vi "2D scan tiled.vi"(11 "Tiled scan inputs":T6={"HW Config"={"SEM X coil"="SEM-X", "SEM Y coil"="SEM-Y", "Detectors"="Detectors", "Det min (V)"=-10.0, "Det max (V)"=10.0, "Eanable COM"=TRUE, "COM port"="COM1", "Detector FIB-NI auto switch"="FIB/port0/line0", "Machine Type"=0, "Machine ID"="Feiss/Sigma-01-42"}, "Det Info"={"Brightness A"=40.0, "Contrast A"=26.0, "Detector B name"="ESB @ 1.0 kV", "Brightness B"=40.0, "Contrast B"=40.0, "Detector C name"="PMT @ 6.0", "Detector D name"="Detector D"}, "SEM Scan Parameters"={"X size (um)"=20.0, "Y size (um)"=20.0, "X center (um)"=0.0, "Y center (um)"=0.0, "X size (V)"=6.190428211586902, "X size auto"=TRUE, "X stig"=[[0.0]], "Y stig"=[[0.0]], "X aln"=[[0.0]], "Y aln"=[[0.0]], "Scan rate (Hz)"=10000000, "Oversampling"=5, "Oversampling auto"=TRUE, "Frame line rampdown ratio"=0.1, "Pixel size (nm)"=10.0, "WD (mm)"=[[3.0]], "X tiles"=1, "Y tiles"=1, "Overlap (um)"=1.0, "Interlaced"=TRUE, "dX (um)"=[0.0], "dY (um)"=[0.0], "Frames"=1}, "SEM Options"={"GetInfo"=TRUE, "Set Det A para"=TRUE, "Set WD"=FALSE, "Set Mag"=TRUE, "Set stig"=FALSE, "Set aln"=FALSE, "Display"=TRUE, "Save"=TRUE, "8-bit"=TRUE, "Detector A"=TRUE, "Detector B"=FALSE, "Detector C"=FALSE, "Detector D"=FALSE, "Inverse A"=FALSE, "Inverse B"=FALSE, "Inverse C"=FALSE, "Inverse D"=FALSE, "Inverse PNG"=TRUE, "Freeze"=TRUE, "PNG only"=FALSE, "Upload"=FALSE, "Delete after upload"=FALSE}, "Focus Index Options"={"Keep aspect ratio"=FALSE, "Show Focus Index"=TRUE, "Focus Index primary grid center"=TRUE, "X Grids"=[[0]], "Y Grids"=[[0]], "Primary X index"=[[0]], "Primary Y index"=[[0]]}, "File Information"={"File path"=path "E:/Images", "Notes"="", "Save recipe"=FALSE, "Load recipe"=FALSE, "Sample ID"=""}, "Milling para"={"X resolution"=4096, "Y resolution"=125001, "X offset (um)"=0.0, "Y offset (um)"=0.0, "X center (um)"=0.0, "Y center (um)"=0.0, "X size (um)"=250.0, "Y size (um)"=250.0, "UL-Ang"=90.0, "UR-Ang"=90.0, "Line milling time (s)"=5.0, "Z-step (nm)"=2.0, "Lines auto pause"=1, "Auto pause"=FALSE, "Mill from Bottom"=FALSE, "FIB FOV (um)"=500.0, "Auto Profile"=FALSE, "Mill start from Last"=FALSE, "FIB PID on"=FALSE, "FIB PID reset"=TRUE, "FIB PID measured"=0, "FIB PID target"=0.0, "FIB PID target slope"=0.0, "FIB PID P"=0.001, "FIB PID I"=0.01, "FIB PID D"=0.0, "Emission (uA)"=1.36, "Suppressor (V)"=50.0, "Auto reheat"=FALSE}} {"Milling para"."Suppressor (V)" step=0.1 format="%.1g"; "Milling para"."Emission (uA)" step=0.1 format="%.2g"; "Milling para"."FIB PID measured" items=["Spec.", "B.D. 1", "B.D. 2", "Mill", "Spec. +"]; "Milling para"."FIB PID target slope" min=-1 max=1 step=0.1; "Milling para"."UR-Ang" format="%.2f"; "Milling para"."UL-Ang" format="%.2f"; "Milling para"."Y offset (um)" step=0.02 format="%.3g"; "Milling para"."X offset (um)" step=1 format="%.3g"; "Milling para"."FIB FOV (um)" format="%.3g"; "Milling para"."Line milling time (s)" format="%.1f"; "Milling para"."Y center (um)" format="%#.3g"; "Milling para"."X center (um)" format="%#.3g"; "SEM Scan Parameters"."dY (um)" format="%.1f"; "SEM Scan Parameters"."dX (um)" format="%.1f"; "SEM Scan Parameters"."Frames" min=1 step=1; "SEM Scan Parameters"."WD (mm)" format="%.1f"; "SEM Scan Parameters"."Y aln" format="%.1f"; "SEM Scan Parameters"."X aln" format="%.1f"; "SEM Scan Parameters"."Y stig" format="%.1f"; "SEM Scan Parameters"."X stig" format="%.1f"; "SEM Scan Parameters"."Overlap (um)" min=0; "SEM Scan Parameters"."Y tiles" min=1; "SEM Scan Parameters"."X tiles" min=1; "SEM Scan Parameters"."X size (um)" format="%.2f"; "SEM Scan Parameters"."Y size (um)" format="%.2f"; "SEM Scan Parameters"."Frame line rampdown ratio" min=0 max=1 step=0.05 format="%.2g"; "SEM Scan Parameters"."X center (um)" step=1 format="%.2f"; "SEM Scan Parameters"."Y center (um)" step=1 format="%.2f"; "SEM Scan Parameters"."X size (V)" format="%_4g"; "SEM Scan Parameters"."Scan rate (Hz)" max=4000000 step=100000 format="%.2e"; "HW Config"."Machine Type" items=["Feiss", "NVision"]}) -> (0 "Image Focus Index Tiled":T3, 1 "Image Focus Index Array Tiled":T2, 2 "Low res scale Tiled (um/pix)":dbl[][](array[numeric]), 3 "Single scan outputs":T4={"SEM Status"={"AO SampClk.MaxRate"=100000000.0, "AI SampClk.MaxRate"=100000000.0, "AO rate"=10000000.0, "Scan speed"=1, "Detector #"=1, "X min (V)"=-3.095214105793451, "X max (V)"=3.095214105793451, "X min index"=0, "X max index"=1999, "AO multiline"=64, "Decimating factor"=3, "AvailSampPerChan"=832704, "AO scan line"=2000, "Total pixels recorded"=4096000, "Lines scanned"=2000, "Scan time (m)"=0.0, "Scan time (s)"=0.4416, "Remaining time (m)"=0, "Remaining time (s)"=0, "SEM Spec. I (nA)"=0.0, "Frame"=1, "X tile"=1, "Y tile"=1}, "SEM Parameters"={"Detector A"="InLens", "Detector B"="ESB @ 1.0 kV", "Brightness A"=40.0, "Contrast A"=26.0, "Brightness B"=40.0, "Contrast B"=40.0, "Magnification"=1769.4047, "Pixel size"=3.9210947, "Working distance"=2.91745, "EHT"=0.6, "Aperture"=1, "High current mode"=1, "Probe current"=613.0, "Scan rotation"=260.0, "Chamber vac"=1.43287e-06, "Gun vac"=3.9272e-10, "Beam shift X"=0.0, "Beam shift Y"=0.0, "Stig X"=-4.213583, "Stig Y"=-1.875912, "Alignment X"=1.861752, "Alignment Y"=-2.407838, "Stage X"=68.4182, "Stage Y"=64.91782, "Stage Z"=32.8349, "Stage T"=0.0, "Stage R"=153.14406, "Stage M"=0.0}, "Image Focus Index"={"A Img Focus Index"=0.014358657, "B Img Focus Index"=0.0, "C Img Focus Index"=0.0, "D Img Focus Index"=0.0}, "FIB parameters"={"FIB mode"=0, "FIB focus"=0.0, "FIB probe current"=0.0, "FIB emission current"=0.0, "FIB rotation"=0.0, "FIB aperture X"=0.0, "FIB aperture Y"=0.0, "FIB stig X"=0.0, "FIB stig Y"=0.0, "FIB beam shift X"=0.0, "FIB beam shift Y"=0.0}, "Image Focus Index Array"={"A Img Focus Index array"=[[0.014358657]], "B Img Focus Index array"=[], "C Img Focus Index array"=[], "D Img Focus Index array"=[]}} {"SEM Status"."Frame" min=1 step=1; "SEM Status"."Y tile" min=1; "SEM Status"."X tile" min=1; "SEM Status"."SEM Spec. I (nA)" format="%.2g"; "SEM Status"."AvailSampPerChan" scale=0.0..32000000.0; "SEM Status"."Scan time (s)" format="%.3f"; "SEM Status"."Total pixels recorded" scale=-1.0..37748736.0; "SEM Status"."Scan speed" scale=1.0..15.0; "SEM Status"."AO rate" format="%#_3e"}, 4 "SEM Spec. I Tiled (nA)":sgl[][](array[numeric]), 5 "8-bit over scale":bool[](array[boolean]))   [LabVIEW 2018]
uses:
  <vilib>/Analysis/baseanly.llb/Mean (DBL).vi
  <vilib>/Analysis/NI_AALBase.lvlib
panel:
  in  "Focus Index Options":T1={"Keep aspect ratio"=FALSE, "X Grids"=1, "Y Grids"=1, "Primary X index"=0, "Primary Y index"=0}
  in  "Api":refnum<k7>(container)
  out "Aln X Tiled":sgl[][](array[numeric])
  out "Aln Y Tiled":sgl[][](array[numeric])
  out "Stig Y Tiled":sgl[][](array[numeric])
  out "Stig X Tiled":sgl[][](array[numeric])
  out "WD Tiled":sgl[][](array[numeric])
  out "Det B Img Tiled":i16[][](graph)
  out "Det A Img Tiled":i16[][](graph)
  out "Tiled image Y index":u16[][](array[numeric])
  out "Tiled image X index":u16[][](array[numeric])
  out "Tiled image scale (um/pix)":sgl
  out "X size (V)":dbl[][](array[numeric])=[[2000.0]]
  out "Y center (um)":sgl[][](array[numeric])
  out "X center (um)":sgl[][](array[numeric])
  out "Y resolution":u32[][](array[numeric])=[[2000]]
  out "X resolution":u32[][](array[numeric])=[[2000]]
  in  "SEM Scan Parameters":T5={"X resolution"=6144, "Y resolution"=6144, "X center (um)"=0.0, "Y center (um)"=0.0, "X size (V)"=6.190428211586902, "X size auto"=TRUE, "X stig"=0.0, "Y stig"=0.0, "X aln"=0.0, "Y aln"=0.0, "Scan rate (Hz)"=10000000, "Oversampling"=5, "Oversampling auto"=TRUE, "Frame line rampdown ratio"=0.1, "Pixel size (nm)"=10.0, "WD (mm)"=0.0} {"Y aln" step=0.2 format="%.1g"; "X aln" step=0.2 format="%.1g"; "Y stig" step=0.2 format="%.1g"; "X stig" step=0.2 format="%.1g"; "WD (mm)" step=0.001 format="%.6g"; "Frame line rampdown ratio" min=0 max=1 step=0.05 format="%.2g"; "X center (um)" step=1.0 format="%.2f"; "Y center (um)" step=1.0 format="%.2f"; "X size (V)" format="%_4g"; "Scan rate (Hz)" max=4000000 step=100000 format="%.2e"}
  # "Hz"
  # "Scanning time"
  # "m"
  # "s"
  # "Remaining time"
  # "m"
  # "s"
  # "Direction"
  # "Start\nfrom"
  # "<"
  # "Grids"
  # "Primary"
  # "Recipe"
  # "Det"
  # "after"
  # "Detector A"
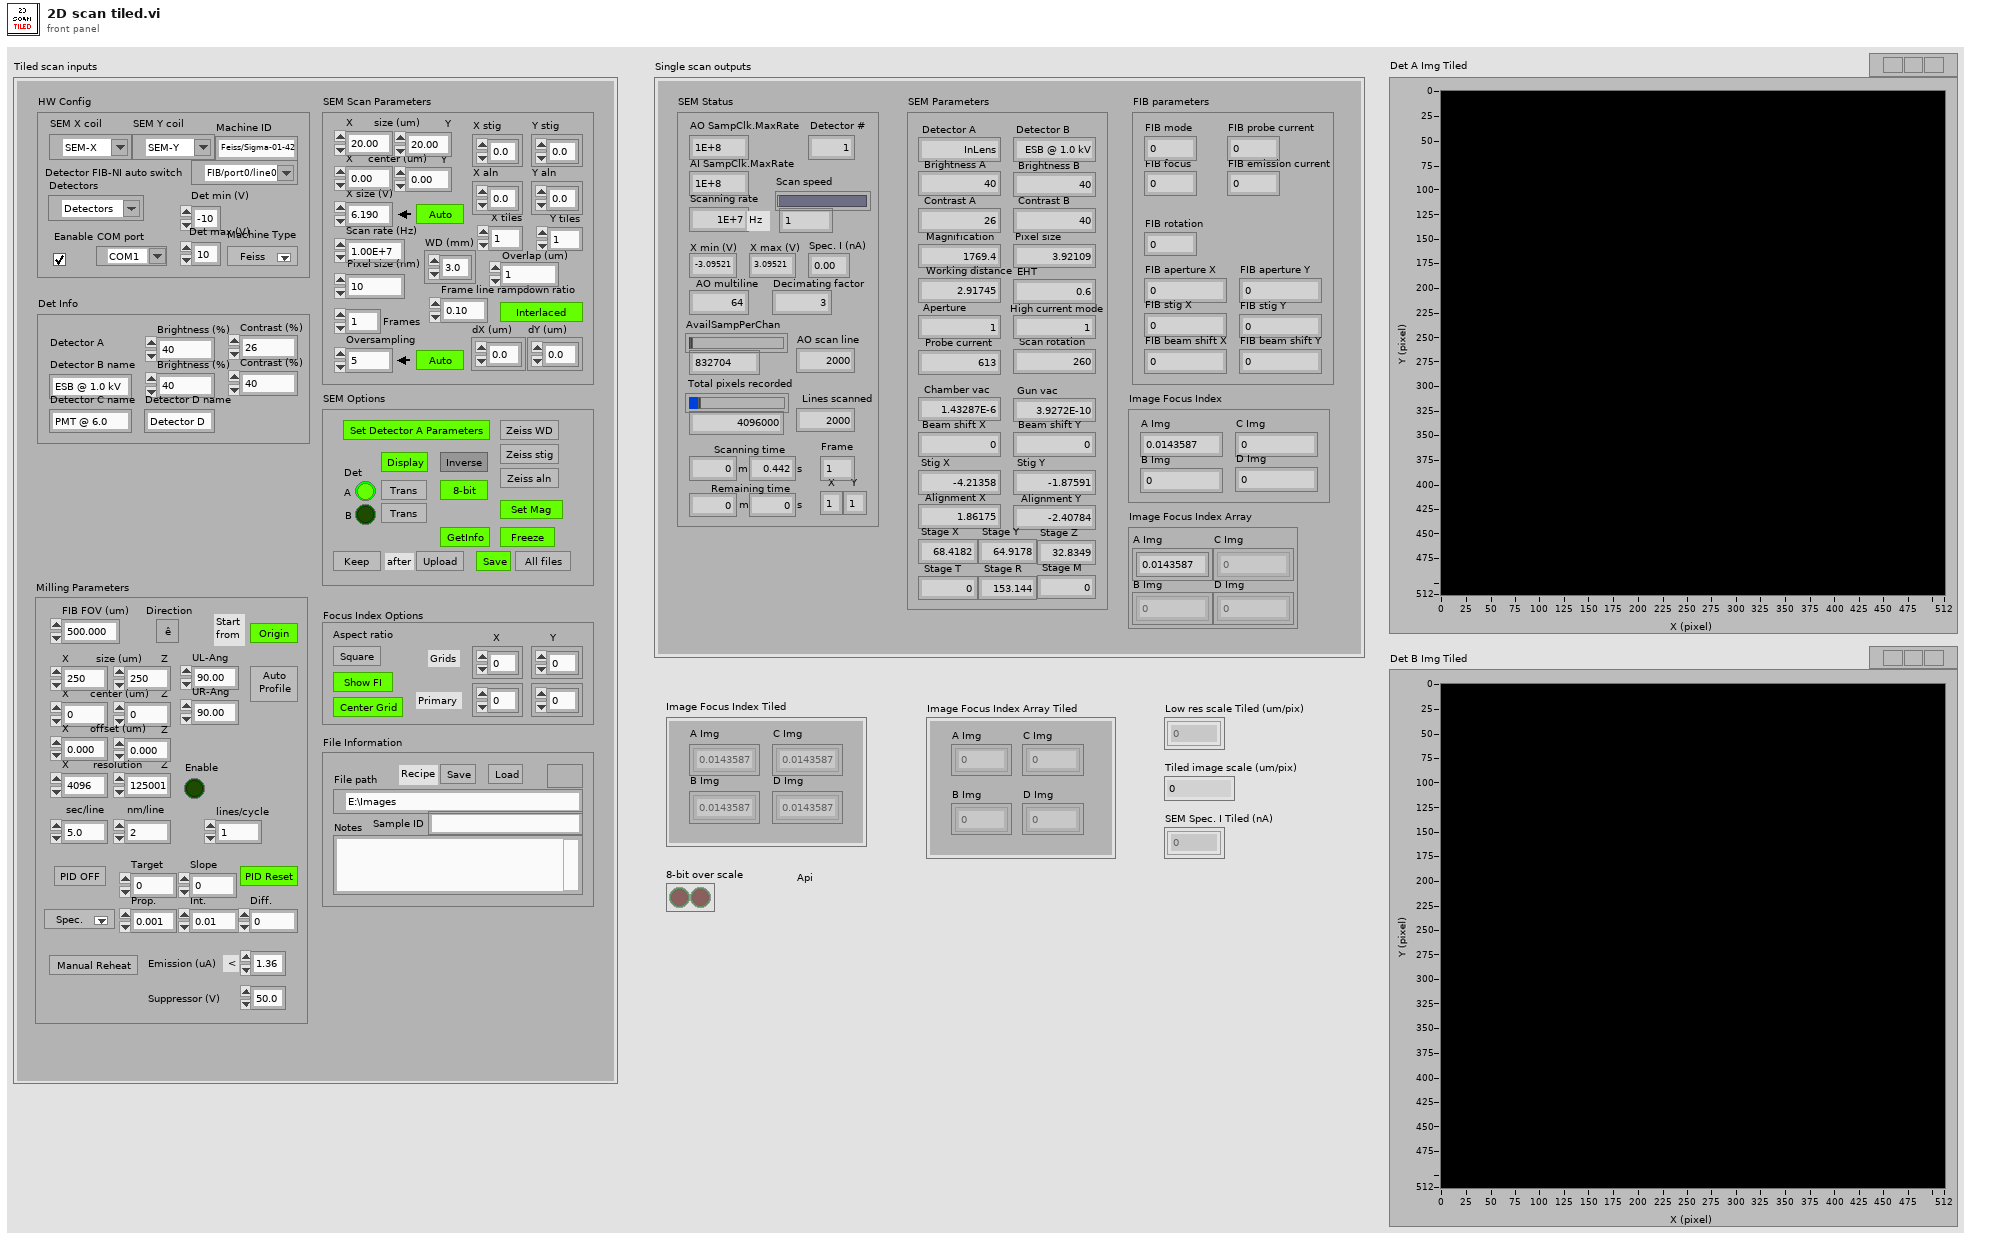
[diagram p1: front panel]
types:
  T1 = cluster{"Keep aspect ratio":bool, "X Grids":u8, "Y Grids":u8, "Primary X index":u8, "Primary Y index":u8}
  T2 = cluster{"A Img Focus Index array":sgl[][][][], "B Img Focus Index array":sgl[][][][], "C Img Focus Index array":sgl[][][][], "D Img Focus Index array":sgl[][][][]}
  T3 = cluster{"A Img Focus Index":sgl[][], "B Img Focus Index":sgl[][], "C Img Focus Index":sgl[][], "D Img Focus Index":sgl[][]}
  T4 = cluster{"SEM Status":cluster{"AO SampClk.MaxRate":dbl, "AI SampClk.MaxRate":dbl, "AO rate":dbl, "Scan speed":u8, "Detector #":u8, "X min (V)":dbl, "X max (V)":dbl, "X min index":i32, "X max index":i32, "AO multiline":u32, "Decimating factor":u16, "AvailSampPerChan":u32, "AO scan line":u32, "Total pixels recorded":i32, "Lines scanned":i32, "Scan time (m)":dbl, "Scan time (s)":dbl, "Remaining time (m)":u16, "Remaining time (s)":u8, "SEM Spec. I (nA)":sgl, "Frame":u8, "X tile":u8, "Y tile":u8}, "SEM Parameters":cluster{"Detector A":string, "Detector B":string, "Brightness A":sgl, "Contrast A":sgl, "Brightness B":sgl, "Contrast B":sgl, "Magnification":sgl, "Pixel size":sgl, "Working distance":sgl, "EHT":sgl, "Aperture":u8, "High current mode":u8, "Probe current":sgl, "Scan rotation":sgl, "Chamber vac":sgl, "Gun vac":sgl, "Beam shift X":sgl, "Beam shift Y":sgl, "Stig X":sgl, "Stig Y":sgl, "Alignment X":sgl, "Alignment Y":sgl, "Stage X":sgl, "Stage Y":sgl, "Stage Z":sgl, "Stage T":sgl, "Stage R":sgl, "Stage M":sgl}, "Image Focus Index":cluster{"A Img Focus Index":sgl, "B Img Focus Index":sgl, "C Img Focus Index":sgl, "D Img Focus Index":sgl}, "FIB parameters":cluster{"FIB mode":u8, "FIB focus":sgl, "FIB probe current":sgl, "FIB emission current":sgl, "FIB rotation":sgl, "FIB aperture X":sgl, "FIB aperture Y":sgl, "FIB stig X":sgl, "FIB stig Y":sgl, "FIB beam shift X":sgl, "FIB beam shift Y":sgl}, "Image Focus Index Array":cluster{"A Img Focus Index array":sgl[][], "B Img Focus Index array":sgl[][], "C Img Focus Index array":sgl[][], "D Img Focus Index array":sgl[][]}}
  T5 = cluster{"X resolution":u32, "Y resolution":u32, "X center (um)":dbl, "Y center (um)":dbl, "X size (V)":dbl, "X size auto":bool, "X stig":sgl, "Y stig":sgl, "X aln":sgl, "Y aln":sgl, "Scan rate (Hz)":u32, "Oversampling":u32, "Oversampling auto":bool, "Frame line rampdown ratio":sgl, "Pixel size (nm)":sgl, "WD (mm)":sgl}
  T6 = cluster{"HW Config":cluster{"SEM X coil":refnum<k15>, "SEM Y coil":refnum<k15>, "Detectors":refnum<k15>, "Det min (V)":dbl, "Det max (V)":dbl, "Eanable COM":bool, "COM port":refnum<visa-resource-name>, "Detector FIB-NI auto switch":tag, "Machine Type":u8, "Machine ID":string}, "Det Info":cluster{"Brightness A":dbl, "Contrast A":dbl, "Detector B name":string, "Brightness B":dbl, "Contrast B":dbl, "Detector C name":string, "Detector D name":string}, "SEM Scan Parameters":cluster{"X size (um)":sgl, "Y size (um)":sgl, "X center (um)":sgl, "Y center (um)":sgl, "X size (V)":dbl, "X size auto":bool, "X stig":sgl[][], "Y stig":sgl[][], "X aln":sgl[][], "Y aln":sgl[][], "Scan rate (Hz)":u32, "Oversampling":u32, "Oversampling auto":bool, "Frame line rampdown ratio":sgl, "Pixel size (nm)":sgl, "WD (mm)":sgl[][], "X tiles":u8, "Y tiles":u8, "Overlap (um)":sgl, "Interlaced":bool, "dX (um)":sgl[], "dY (um)":sgl[], "Frames":u8}, "SEM Options":cluster{"GetInfo":bool, "Set Det A para":bool, "Set WD":bool, "Set Mag":bool, "Set stig":bool, "Set aln":bool, "Display":bool, "Save":bool, "8-bit":bool, "Detector A":bool, "Detector B":bool, "Detector C":bool, "Detector D":bool, "Inverse A":bool, "Inverse B":bool, "Inverse C":bool, "Inverse D":bool, "Inverse PNG":bool, "Freeze":bool, "PNG only":bool, "Upload":bool, "Delete after upload":bool}, "Focus Index Options":cluster{"Keep aspect ratio":bool, "Show Focus Index":bool, "Focus Index primary grid center":bool, "X Grids":u8[][], "Y Grids":u8[][], "Primary X index":u8[][], "Primary Y index":u8[][]}, "File Information":cluster{"File path":path, "Notes":string, "Save recipe":bool, "Load recipe":bool, "Sample ID":string}, "Milling para":cluster{"X resolution":u32, "Y resolution":u32, "X offset (um)":sgl, "Y offset (um)":sgl, "X center (um)":sgl, "Y center (um)":sgl, "X size (um)":sgl, "Y size (um)":sgl, "UL-Ang":sgl, "UR-Ang":sgl, "Line milling time (s)":sgl, "Z-step (nm)":dbl, "Lines auto pause":u16, "Auto pause":bool, "Mill from Bottom":bool, "FIB FOV (um)":sgl, "Auto Profile":bool, "Mill start from Last":bool, "FIB PID on":bool, "FIB PID reset":bool, "FIB PID measured":u8, "FIB PID target":sgl, "FIB PID target slope":sgl, "FIB PID P":sgl, "FIB PID I":sgl, "FIB PID D":sgl, "Emission (uA)":dbl, "Suppressor (V)":sgl, "Auto reheat":bool}}
  T7 = cluster{"GetInfo":bool, "Set Det A para":bool, "Set WD":bool, "Set Mag":bool, "Set stig":bool, "Set aln":bool, "Display":bool, "Save":bool, "8-bit":bool, "Detector A":bool, "Detector B":bool, "Detector C":bool, "Detector D":bool, "Inverse A":bool, "Inverse B":bool, "Inverse C":bool, "Inverse D":bool, "Inverse PNG":bool, "Freeze":bool, "PNG only":bool, "Upload":bool, "Delete after upload":bool}
  T8 = cluster{"SEM X coil":refnum<k15>, "SEM Y coil":refnum<k15>, "Detectors":refnum<k15>, "Det min (V)":dbl, "Det max (V)":dbl, "Eanable COM":bool, "COM port":refnum<visa-resource-name>, "Detector FIB-NI auto switch":tag, "Machine Type":u8, "Machine ID":string}
  T9 = cluster{"Brightness A":dbl, "Contrast A":dbl, "Detector B name":string, "Brightness B":dbl, "Contrast B":dbl, "Detector C name":string, "Detector D name":string}
  T10 = cluster{"X size (um)":sgl, "Y size (um)":sgl, "X center (um)":sgl, "Y center (um)":sgl, "X size (V)":dbl, "X size auto":bool, "X stig":sgl[][], "Y stig":sgl[][], "X aln":sgl[][], "Y aln":sgl[][], "Scan rate (Hz)":u32, "Oversampling":u32, "Oversampling auto":bool, "Frame line rampdown ratio":sgl, "Pixel size (nm)":sgl, "WD (mm)":sgl[][], "X tiles":u8, "Y tiles":u8, "Overlap (um)":sgl, "Interlaced":bool, "dX (um)":sgl[], "dY (um)":sgl[], "Frames":u8}
  T11 = cluster{"Keep aspect ratio":bool, "Show Focus Index":bool, "Focus Index primary grid center":bool, "X Grids":u8[][], "Y Grids":u8[][], "Primary X index":u8[][], "Primary Y index":u8[][]}
  T12 = cluster{"File path":path, "Notes":string, "Save recipe":bool, "Load recipe":bool, "Sample ID":string}
  T13 = cluster{"X resolution":u32, "Y resolution":u32, "X offset (um)":sgl, "Y offset (um)":sgl, "X center (um)":sgl, "Y center (um)":sgl, "X size (um)":sgl, "Y size (um)":sgl, "UL-Ang":sgl, "UR-Ang":sgl, "Line milling time (s)":sgl, "Z-step (nm)":dbl, "Lines auto pause":u16, "Auto pause":bool, "Mill from Bottom":bool, "FIB FOV (um)":sgl, "Auto Profile":bool, "Mill start from Last":bool, "FIB PID on":bool, "FIB PID reset":bool, "FIB PID measured":u8, "FIB PID target":sgl, "FIB PID target slope":sgl, "FIB PID P":sgl, "FIB PID I":sgl, "FIB PID D":sgl, "Emission (uA)":dbl, "Suppressor (V)":sgl, "Auto reheat":bool}
  T14 = cluster{"A Img Focus Index array":sgl[][], "B Img Focus Index array":sgl[][], "C Img Focus Index array":sgl[][], "D Img Focus Index array":sgl[][]}
  T15 = cluster{"AO SampClk.MaxRate":dbl, "AI SampClk.MaxRate":dbl, "AO rate":dbl, "Scan speed":u8, "Detector number":u8, "X min (V)":dbl, "X max (V)":dbl, "X min index":i32, "X max index":i32, "AO multiline":u32, "Decimating factor":u16, "AvailSampPerChan":u32, "AO scan line":u32, "Total pixels recorded":i32, "Total lines scanned":i32, "Scan time (m)":dbl, "Scan time (s)":dbl, "Remaining time (m)":u16, "Remaining time (s)":u8, "Specimen I (nA)":sgl, "Frame":u8, "X tile":u8, "Y tile":u8}
  T16 = cluster{"Detector A":string, "Detector B":string, "Brightness A":sgl, "Contrast A":sgl, "Brightness B":sgl, "Contrast B":sgl, "Magnification":sgl, "Pixel size":sgl, "Working distance":sgl, "EHT":sgl, "Aperture":u8, "High current mode":u8, "Probe current":sgl, "Scan rotation":sgl, "Chamber vac":sgl, "Gun vac":sgl, "Beam shift X":sgl, "Beam shift Y":sgl, "Stig X":sgl, "Stig Y":sgl, "Alignment X":sgl, "Alignment Y":sgl, "Stage X":sgl, "Stage Y":sgl, "Stage Z":sgl, "Stage T":sgl, "Stage R":sgl, "Stage M":sgl}
  T17 = cluster{"FIB mode":u8, "FIB focus":sgl, "FIB probe current":sgl, "FIB emission current":sgl, "FIB rotation":sgl, "FIB aperture X":sgl, "FIB aperture Y":sgl, "FIB stig X":sgl, "FIB stig Y":sgl, "FIB beam shift X":sgl, "FIB beam shift Y":sgl}
  T18 = cluster{"A Img Focus Index":sgl, "B Img Focus Index":sgl, "C Img Focus Index":sgl, "D Img Focus Index":sgl}
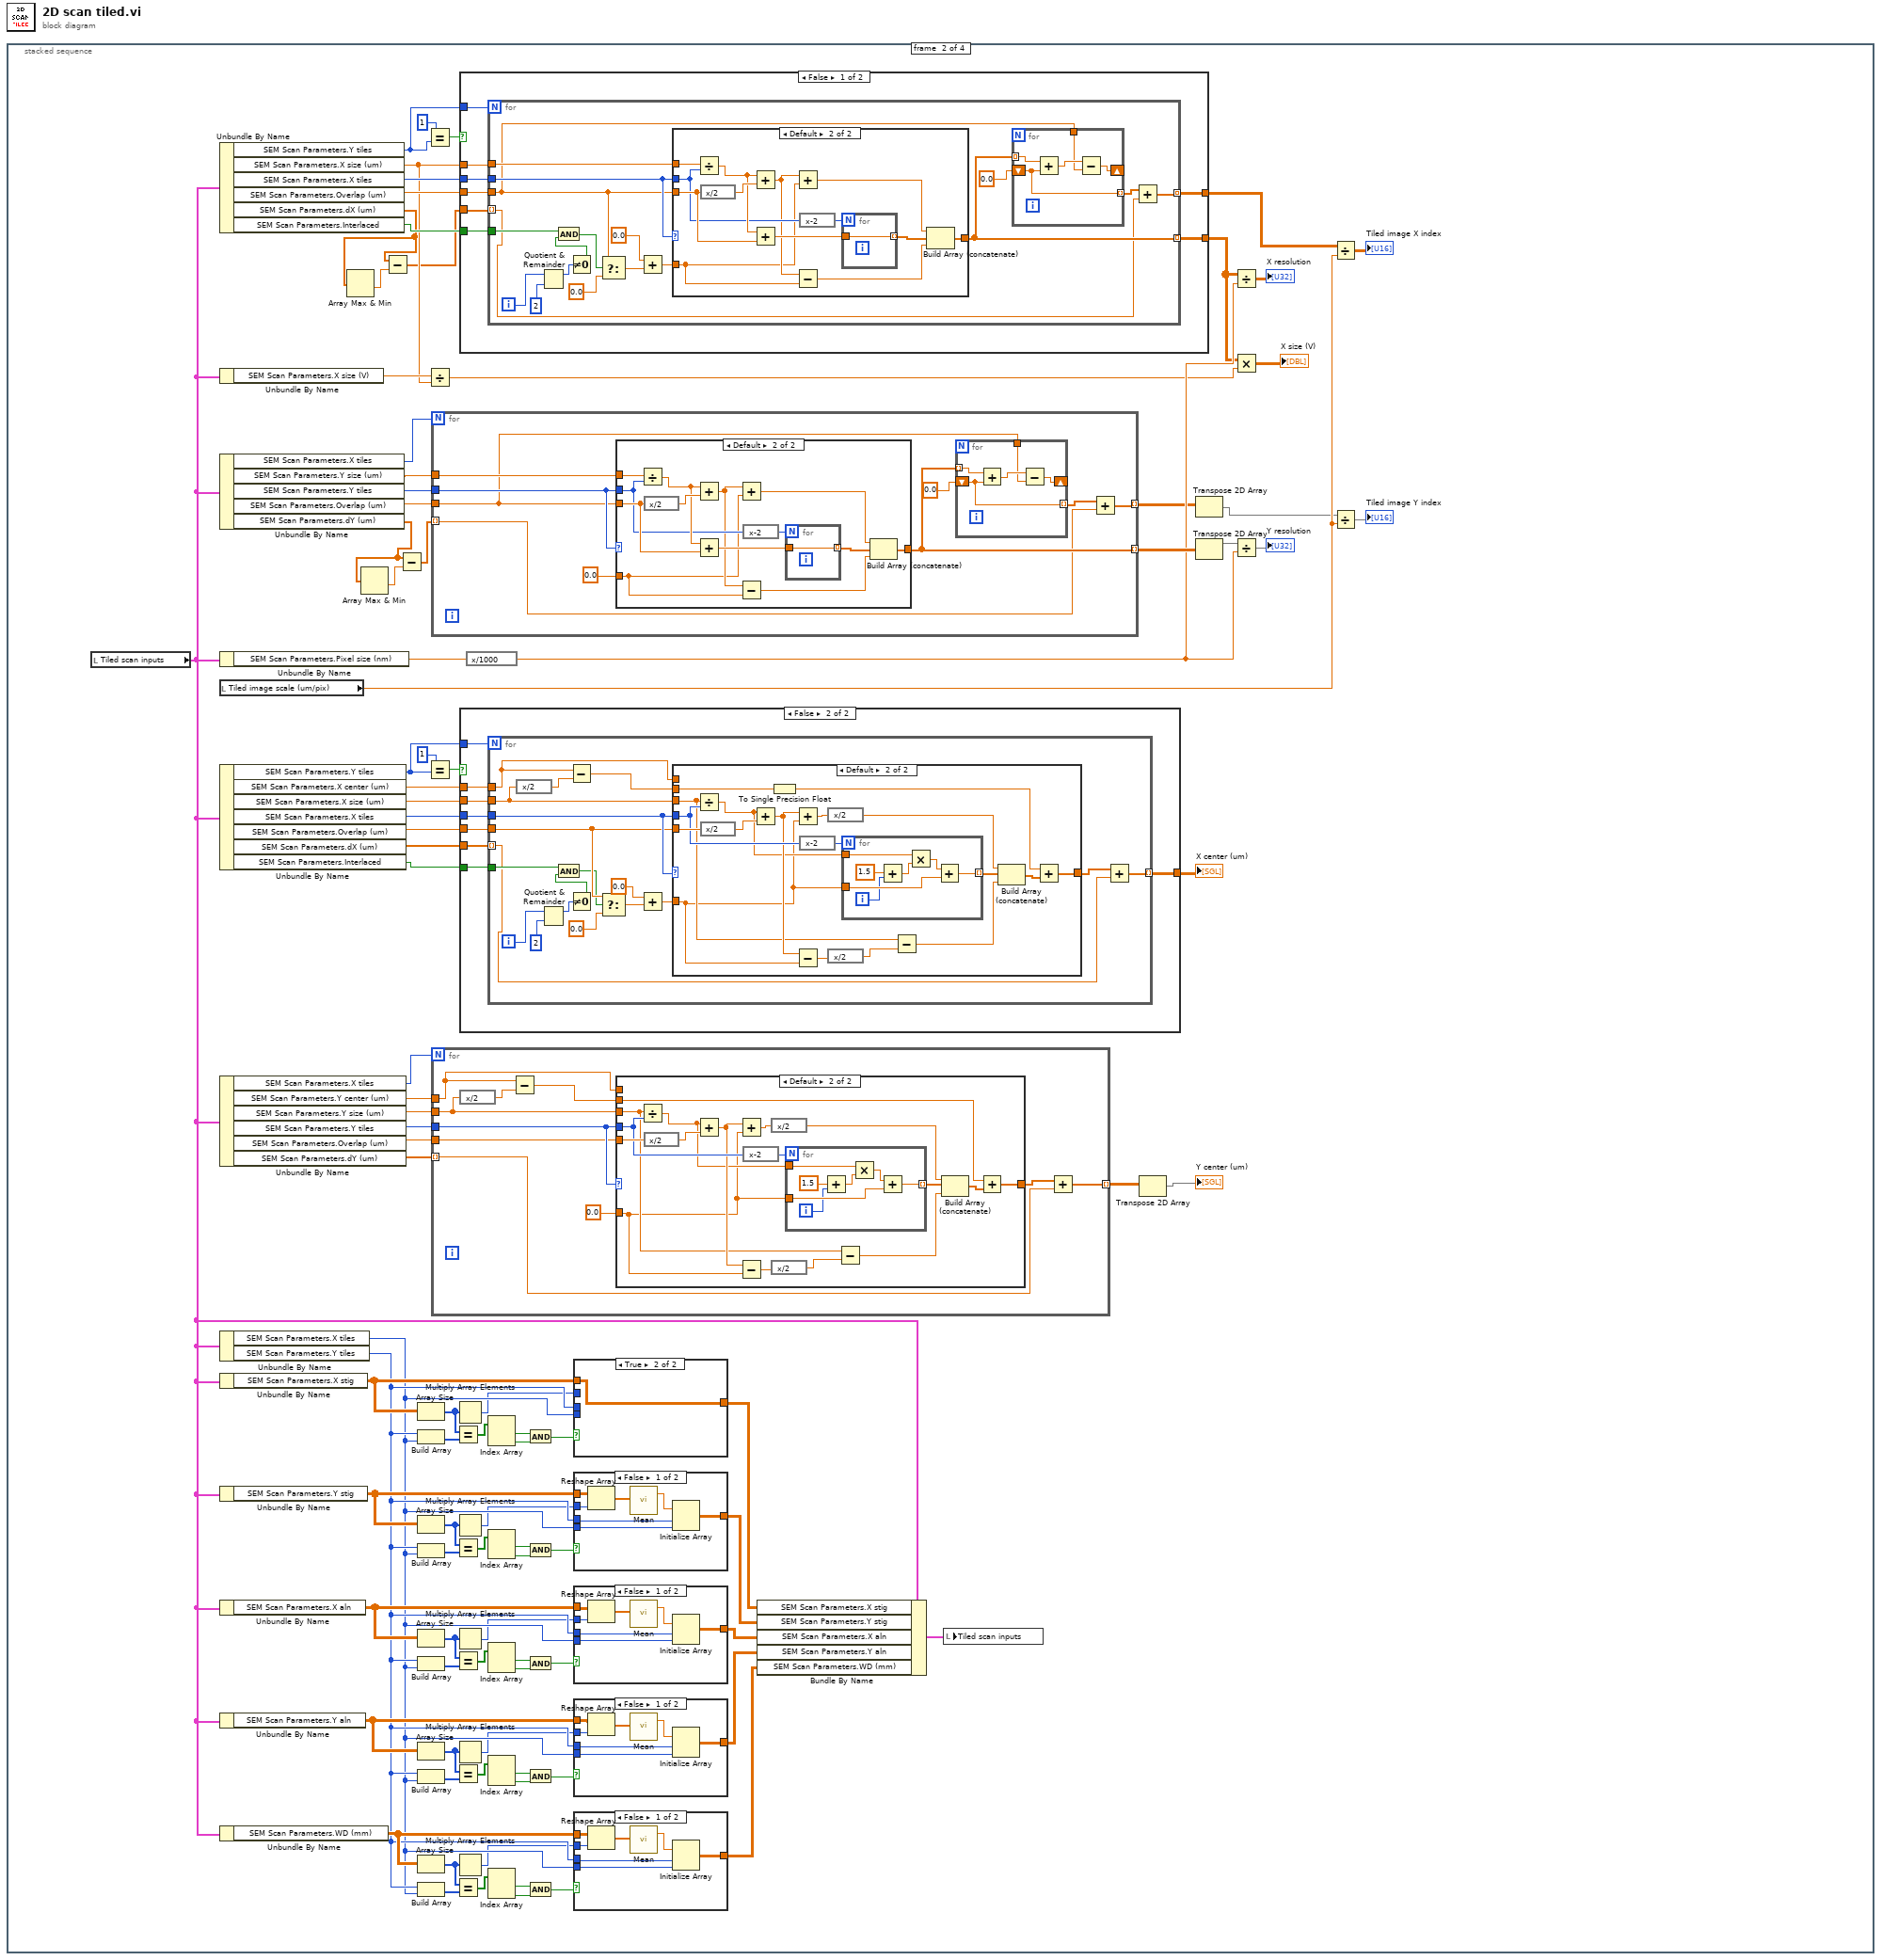
[diagram p0: block diagram]
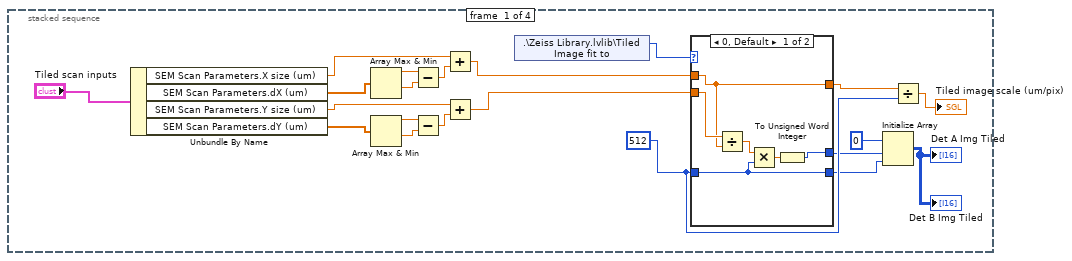
[diagram p2: hidden frame]
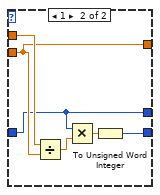
[diagram p3: hidden frame]
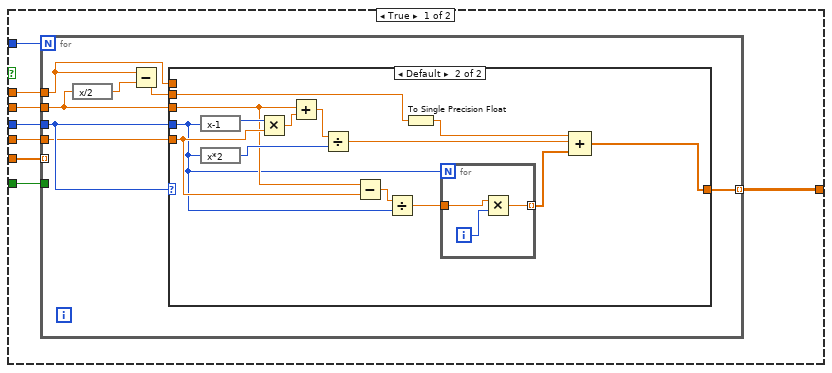
[diagram p4: hidden frame]
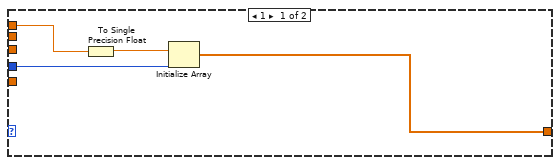
[diagram p5: hidden frame]
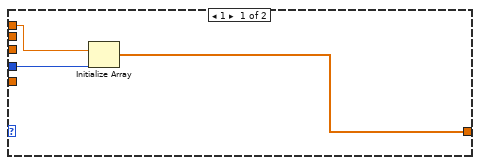
[diagram p6: hidden frame]
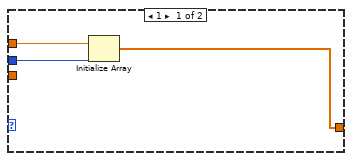
[diagram p7: hidden frame]
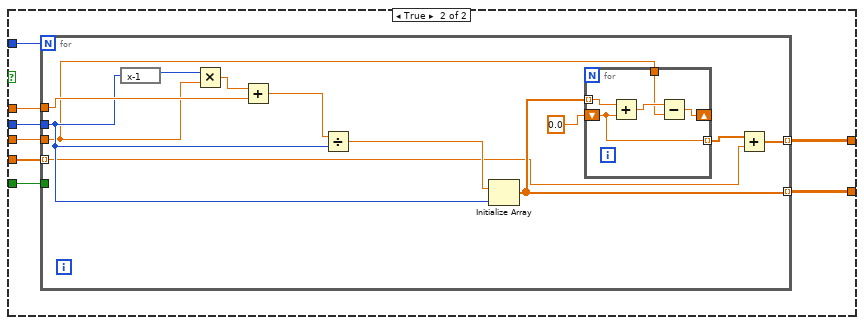
[diagram p8: hidden frame]
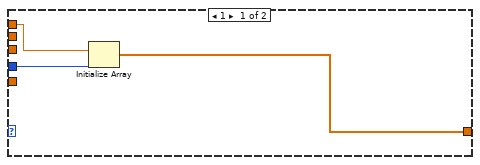
[diagram p9: hidden frame]
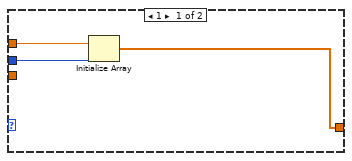
[diagram p10: hidden frame]
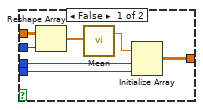
[diagram p15: hidden frame]
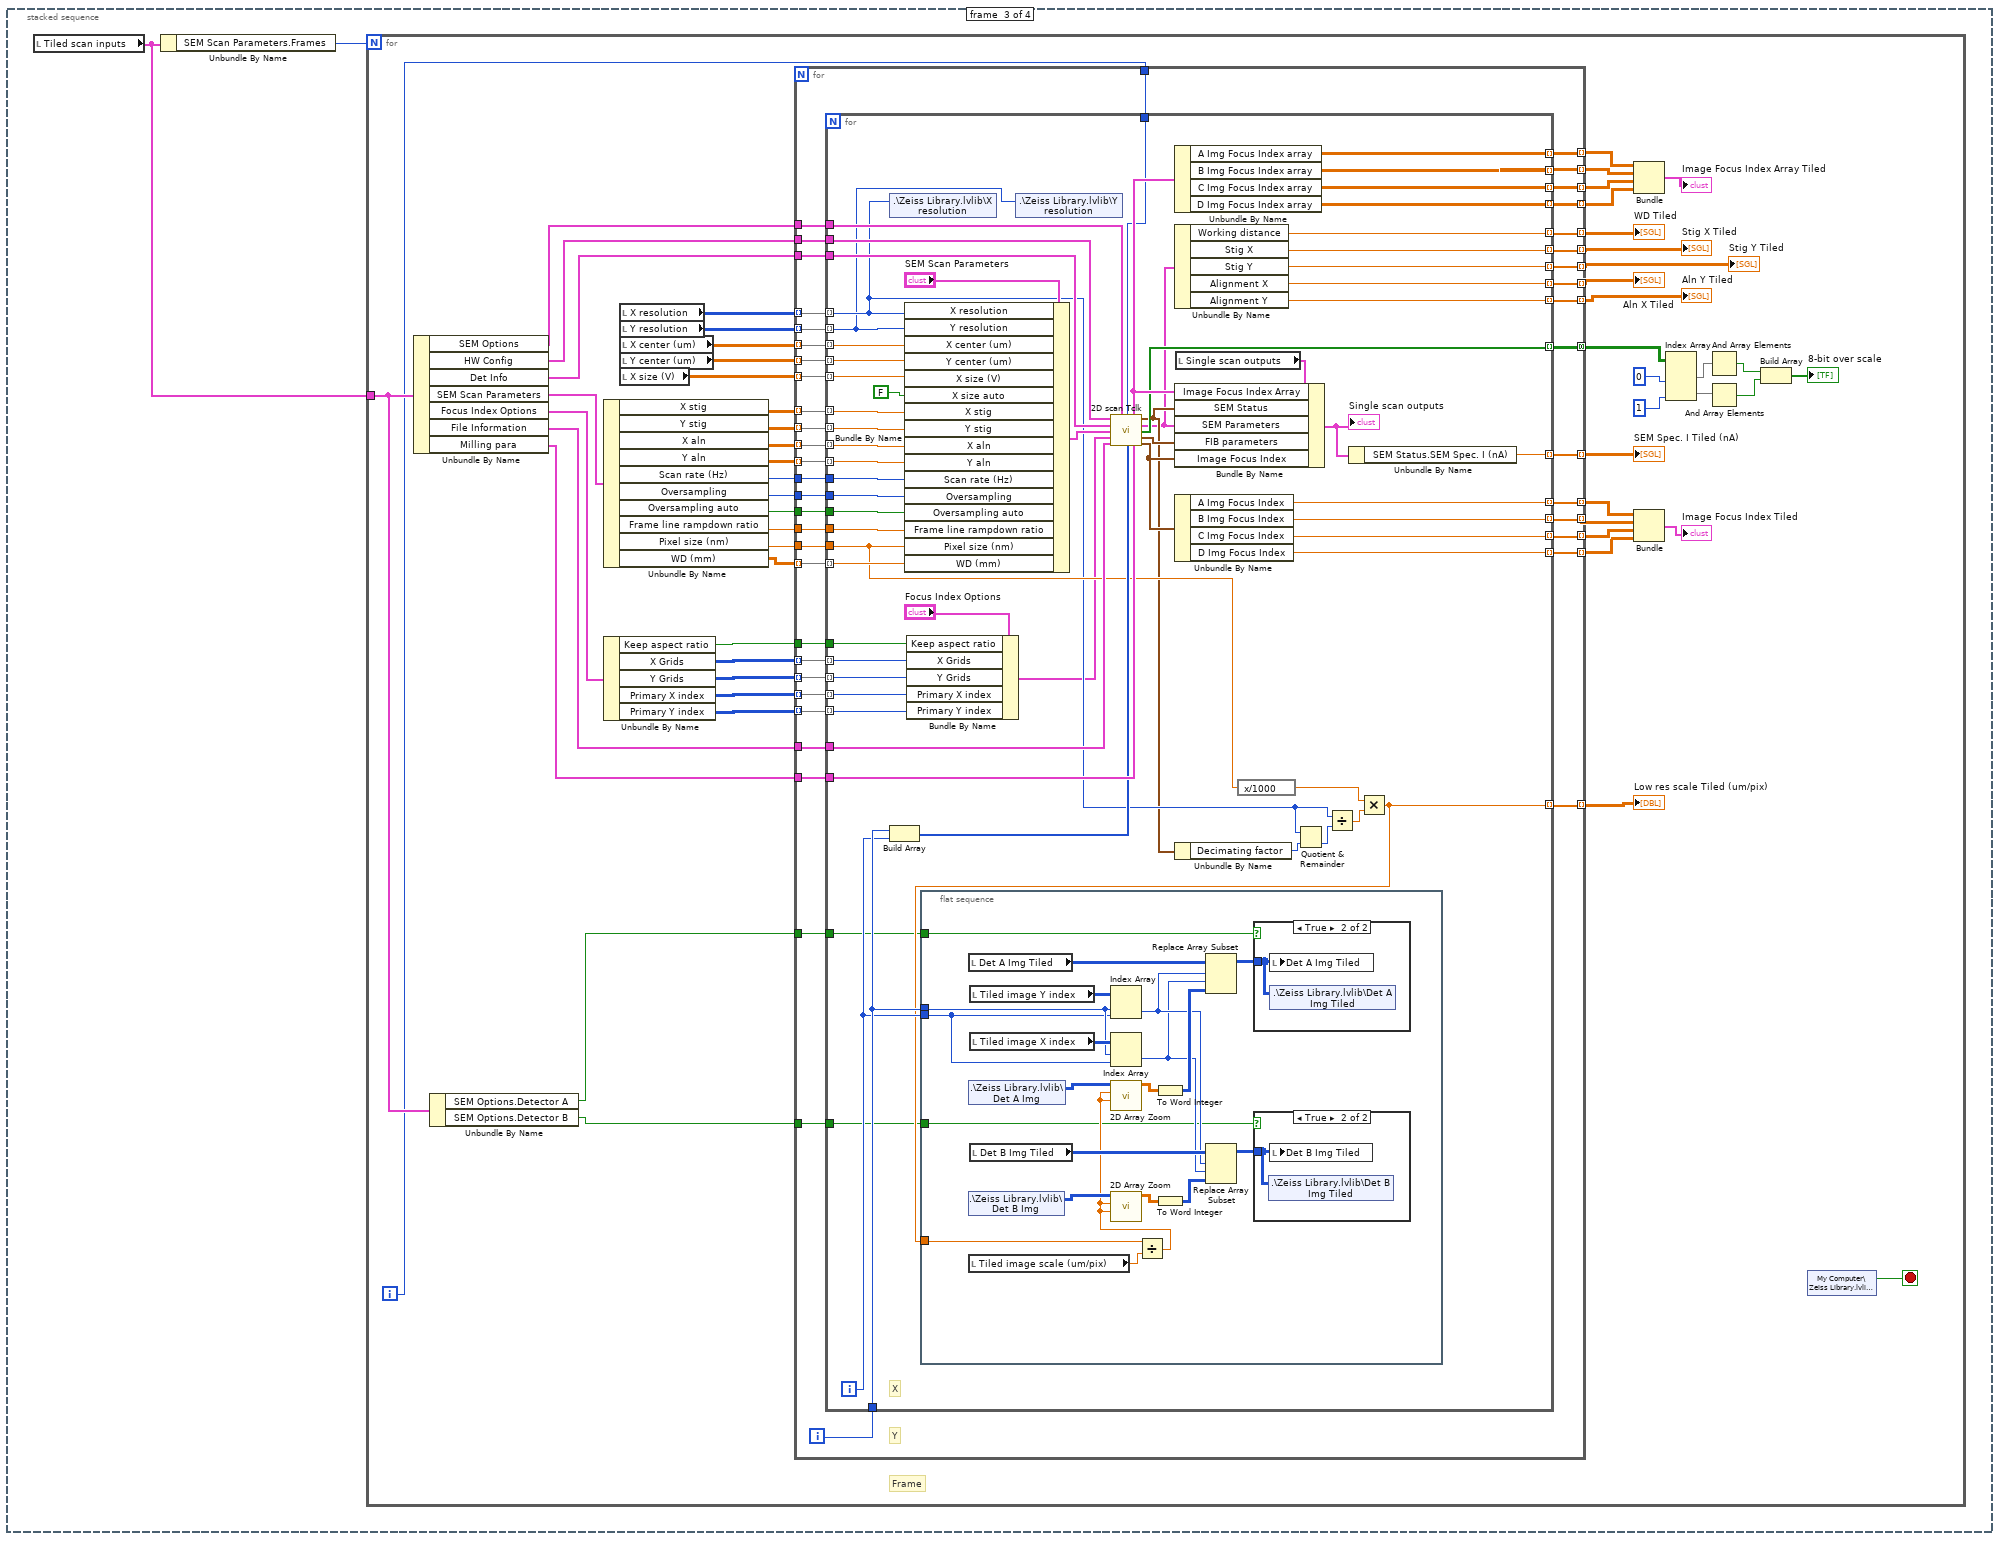
[diagram p16: hidden frame]
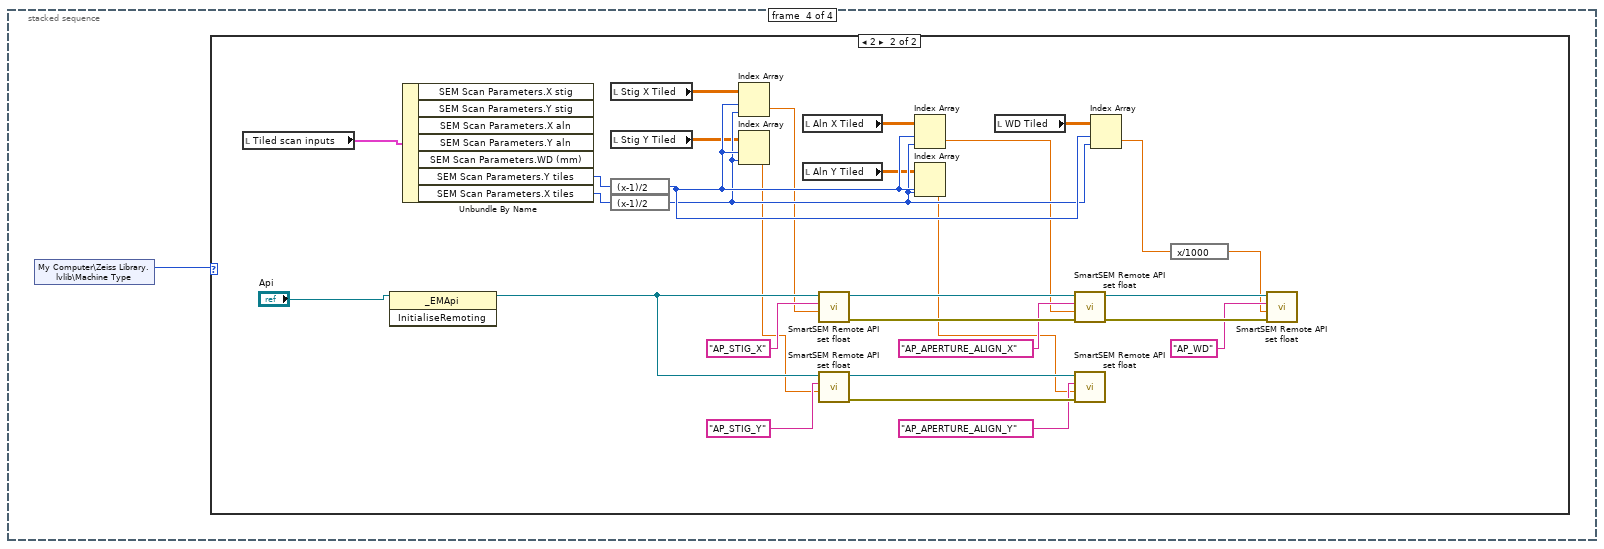
[diagram p19: hidden frame]
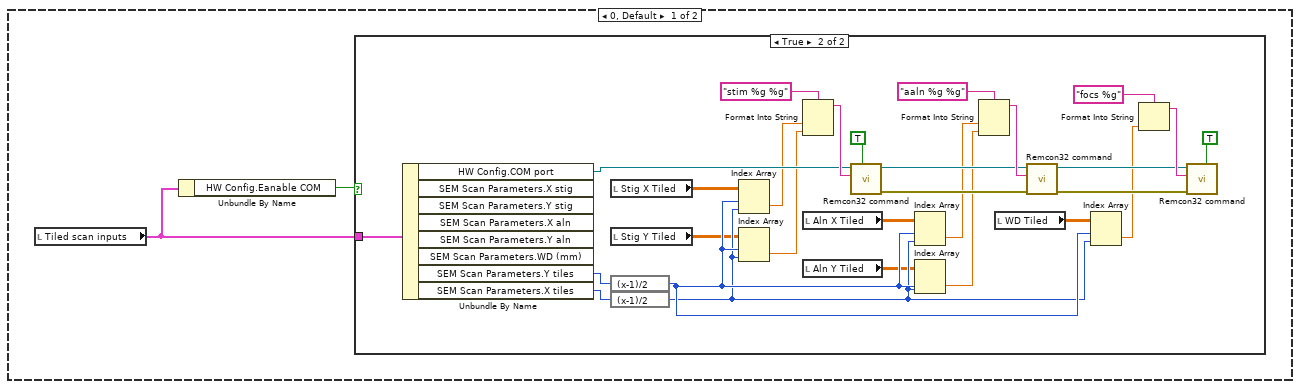
[diagram p20: hidden frame]
diagram:
  n1 = stacked-sequence {
    frame #0 {
      w18 = u16 512 ("y")
      n2 = Unbundle By Name("Tiled scan inputs") -> ("SEM Scan Parameters.X size (um)"=w8:sgl, "SEM Scan Parameters.dX (um)"=w12:sgl[], "SEM Scan Parameters.Y size (um)"=w2:sgl, "SEM Scan Parameters.dY (um)"=w3:sgl[])
      n3 = Array Max & Min(array=w12) -> (max value=w11:sgl, min value=w10:sgl)  [unwired: 2 out]
      n4 = Array Max & Min(array=w3) -> (max value=w4:sgl, min value=w5:sgl)  [unwired: 2 out]
      n5 = Subtract(x=w11, y=w10) -> (x-y=w9:sgl)
      n6 = Subtract(x=w4, y=w5) -> (x-y=w6:sgl)
      n7 = Add(x=w8, y=w9) -> (x+y=w7:sgl)
      n8 = Add(x=w2, y=w6) -> (x+y=w1:sgl)
      n9 = shared-variable ".\\Zeiss Library.lvlib\\Tiled Image fit to"() -> (w13:u8)  [unwired: 1 in, 1 out]
      n10 = case shown="0, Default" w13 {
        tunnel: w7 -> [w26 w32]
        tunnel: w1 -> [w27 w31]
        tunnel: [w26 w31] -> w19
        tunnel: w18 -> [w24 w29]
        tunnel: [w24 w28] -> w16
        tunnel: [w22 w29] -> w17
        frame 0, Default {
          n11 = Divide(x=w27, y=w26) -> (x/y=w25:sgl)
          n12 = Multiply(x=w25, y=w24) -> (x*y=w23:sgl)
          n13 = To Unsigned Word Integer(number=w23) -> (unsigned 16bit integer=w22:u16)
        }
        frame 1 {
          n14 = Divide(x=w32, y=w31) -> (x/y=w30:sgl)
          n15 = Multiply(x=w29, y=w30) -> (x*y=w33:sgl)
          n16 = To Unsigned Word Integer(number=w33) -> (unsigned 16bit integer=w28:u16)
        }
      }
      n17 = Initialize Array(i16 0 ("element"), w17, w16) -> (→"Det A Img Tiled" →"Det B Img Tiled":i16[][])
      n18 = Divide(x=w19, y=w18) -> (x/y=→"Tiled image scale (um/pix)":sgl)
    }
    frame #1 {
      n19 = local read "Tiled scan inputs"() -> (w54:T6)
      n20 = Unbundle By Name(w54) -> ("SEM Scan Parameters.Y tiles"=w44:u8, "SEM Scan Parameters.X size (um)"=w57:sgl, "SEM Scan Parameters.X tiles"=w126:u8, "SEM Scan Parameters.Overlap (um)"=w127:sgl, "SEM Scan Parameters.dX (um)"=w38:sgl[], "SEM Scan Parameters.Interlaced"=w118:bool)
      n21 = Unbundle By Name(w54) -> ("SEM Scan Parameters.X size (V)"=w58:dbl)
      n22 = Unbundle By Name(w54) -> ("SEM Scan Parameters.X tiles"=w120:u8, "SEM Scan Parameters.Y size (um)"=w121:sgl, "SEM Scan Parameters.Y tiles"=w123:u8, "SEM Scan Parameters.Overlap (um)"=w122:sgl, "SEM Scan Parameters.dY (um)"=w34:sgl[])
      n23 = Unbundle By Name(w54) -> ("SEM Scan Parameters.Pixel size (nm)"=w125:sgl)
      n24 = local read "Tiled image scale (um/pix)"() -> (w52:sgl)
      n25 = Unbundle By Name(w54) -> ("SEM Scan Parameters.Y tiles"=w41:u8, "SEM Scan Parameters.X center (um)"=w110:sgl, "SEM Scan Parameters.X size (um)"=w111:sgl, "SEM Scan Parameters.X tiles"=w114:u8, "SEM Scan Parameters.Overlap (um)"=w112:sgl, "SEM Scan Parameters.dX (um)"=w113:sgl[], "SEM Scan Parameters.Interlaced"=w115:bool)
      n26 = Unbundle By Name(w54) -> ("SEM Scan Parameters.X tiles"=w103:u8, "SEM Scan Parameters.Y center (um)"=w108:sgl, "SEM Scan Parameters.Y size (um)"=w107:sgl, "SEM Scan Parameters.Y tiles"=w104:u8, "SEM Scan Parameters.Overlap (um)"=w106:sgl, "SEM Scan Parameters.dY (um)"=w105:sgl[])
      n27 = Unbundle By Name(w54) -> ("SEM Scan Parameters.X tiles"=w72:u8, "SEM Scan Parameters.Y tiles"=w73:u8)
      n28 = Unbundle By Name(w54) -> ("SEM Scan Parameters.X stig"=w133:sgl[][])
      n29 = Unbundle By Name(w54) -> ("SEM Scan Parameters.Y stig"=w90:sgl[][])
      n30 = Unbundle By Name(w54) -> ("SEM Scan Parameters.X aln"=w76:sgl[][])
      n31 = Unbundle By Name(w54) -> ("SEM Scan Parameters.Y aln"=w75:sgl[][])
      n32 = Unbundle By Name(w54) -> ("SEM Scan Parameters.WD (mm)"=w74:sgl[][])
      n33 = Array Max & Min(array=w38) -> (min value=w39:sgl)  [unwired: 3 out]
      n34 = Array Max & Min(array=w34) -> (min value=w36:sgl)  [unwired: 3 out]
      n35 = Subtract(x=w38, y=w39) -> (x-y=w37:sgl[])
      n36 = Subtract(x=w34, y=w36) -> (x-y=w35:sgl[])
      n37 = Array Size(array=w133) -> (size(s)=w68:i32[])
      n38 = Build Array(w73, w72) -> (w99:u8[])
      n39 = Array Size(array=w90) -> (size(s)=w63:i32[])
      n40 = Build Array(w73, w72) -> (w91:u8[])
      n41 = Array Size(array=w76) -> (size(s)=w64:i32[])
      n42 = Build Array(w73, w72) -> (w88:u8[])
      n43 = Array Size(array=w75) -> (size(s)=w66:i32[])
      n44 = Build Array(w73, w72) -> (w81:u8[])
      n45 = Array Size(array=w74) -> (size(s)=w65:i32[])
      n46 = Build Array(w73, w72) -> (w80:u8[])
      n47 = Equal?(x=u8 1, y=w44) -> (x = y?=w45:bool)
      n48 = Divide(x=w58, y=w57) -> (x/y=w56:dbl)
      n49 = Equal?(x=u8 1, y=w41) -> (x = y?=w40:bool)
      n50 = for {
        N: w120 -> [_]
        tunnel: w123 -> [w343]
        tunnel: w122 -> [w339]
        tunnel: w121 -> [w342]
        tunnel: [w340] -> w119 mode=indexing
        tunnel: [w336] -> w47 mode=indexing
        tunnel: w35 -> [w335] mode=indexing
        n51 = case shown="Default" w343 {
          tunnel: w342 -> [w351 w364]
          tunnel: w339 -> [_ w361]
          tunnel: w343 -> [w350 w358]
          tunnel: sgl 0.0 ("element") -> [_ w356]
          tunnel: [w349 w352] -> w340
          frame 1 {
            n52 = Initialize Array(w351, w350) -> (w349:sgl[])
          }
          frame Default {
            n53 = Divide(x=w364, y=w358) -> (x/y=w362:sgl)
            n54 = expression code="x/2"(w361) -> (w363:sgl)
            n55 = Add(x=w362, y=w363) -> (x+y=w357:sgl)
            n56 = Add(x=w362, y=w361) -> (x+y=w360:sgl)
            n57 = Add(x=w357, y=w356) -> (x+y=w355:sgl)
            n58 = Subtract(x=w357, y=w356) -> (x-y=w353:sgl)
            n59 = expression code="x-2"(w358) -> (w359:u8)
            n60 = for {
              N: w359 -> [_]
              tunnel: w360 -> [w365]
              tunnel: [w365] -> w354 mode=indexing
            }
            n61 = Build Array (concatenate)(w355, w354, w353) -> (w352:sgl[])
          }
        }
        n62 = for {
          tunnel: w340 -> [w348] mode=indexing
          shift-right: [w345] -> _
          shift-left: sgl 0.0 -> [w346]
          tunnel: [w346] -> w337 mode=indexing
          tunnel: w339 -> [w344]
          n63 = Add(x=w348, y=w346) -> (x+y=w347:sgl)
          n64 = Subtract(x=w347, y=w344) -> (x-y=w345:sgl)
        }
        n65 = Add(x=w337, y=w335) -> (x+y=w336:sgl[])
      }
      n66 = for {
        N: w103 -> [_]
        tunnel: w107 -> [w305]
        tunnel: w106 -> [w306]
        tunnel: w105 -> [w298] mode=indexing
        tunnel: w104 -> [w307]
        tunnel: [w299] -> w102 mode=indexing
        tunnel: w108 -> [w302]
        n67 = expression code="x/2"(w305) -> (w304:sgl)
        n68 = Subtract(x=w302, y=w304) -> (x-y=w303:sgl)
        n69 = case shown="Default" w307 {
          tunnel: w305 -> [_ w315]
          tunnel: w306 -> [_ w326]
          tunnel: w307 -> [w310 w324]
          tunnel: sgl 0.0 ("element") -> [_ w312]
          tunnel: [w309 w318] -> w300
          tunnel: w303 -> [_ w321]
          tunnel: w302 -> [w308 _]
          frame 1 {
            n70 = Initialize Array(w308, w310) -> (w309:sgl[])
          }
          frame Default {
            n71 = Divide(x=w315, y=w324) -> (x/y=w313:sgl)
            n72 = expression code="x/2"(w326) -> (w327:sgl)
            n73 = Add(x=w313, y=w327) -> (x+y=w323:sgl)
            n74 = Add(x=w323, y=w312) -> (x+y=w322:sgl)
            n75 = Subtract(x=w323, y=w312) -> (x-y=w317:sgl)
            n76 = expression code="x-2"(w324) -> (w325:u8)
            n77 = expression code="x/2"(w322) -> (w320:sgl)
            n78 = expression code="x/2"(w317) -> (w314:sgl)
            n79 = for {
              N: w325 -> [_]
              tunnel: w313 -> [w334]
              tunnel: w312 -> [w332]
              tunnel: [w331] -> w311 mode=indexing
              i -> [w328]
              n80 = Add(x=sgl 1.5, y=w328) -> (x+y=w329:sgl)
              n81 = Multiply(x=w334, y=w329) -> (x*y=w333:sgl)
              n82 = Add(x=w333, y=w332) -> (x+y=w331:sgl)
            }
            n83 = Subtract(x=w315, y=w314) -> (x-y=w316:sgl)
            n84 = Build Array (concatenate)(w320, w311, w316) -> (w319:sgl[])
            n85 = Add(x=w321, y=w319) -> (x+y=w318:sgl[])
          }
        }
        n86 = Add(x=w300, y=w298) -> (x+y=w299:sgl[])
      }
      n87 = Equal?(x=w68, y=w99) -> (x = y?=w98:bool[])
      n88 = Equal?(x=w63, y=w91) -> (x = y?=w92:bool[])
      n89 = Equal?(x=w64, y=w88) -> (x = y?=w87:bool[])
      n90 = Equal?(x=w66, y=w81) -> (x = y?=w82:bool[])
      n91 = Equal?(x=w65, y=w80) -> (x = y?=w79:bool[])
      n92 = Multiply Array Elements(1:w68) -> (0:w67:i32)
      n93 = Multiply Array Elements(1:w63) -> (0:w62:i32)
      n94 = Multiply Array Elements(1:w64) -> (0:w61:i32)
      n95 = Multiply Array Elements(1:w66) -> (0:w60:i32)
      n96 = Multiply Array Elements(1:w65) -> (0:w59:i32)
      n97 = case shown="False" w45 {
        tunnel: w127 -> [w232 w280]
        tunnel: w126 -> [w231 w279]
        tunnel: w44 -> [w230 w278]
        tunnel: w118 -> [w229 w277]
        tunnel: w57 -> [w228 w276]
        tunnel: [w227 w275] -> w49
        tunnel: [w226 w274] -> w48
        tunnel: w37 -> [w225 w273]
        frame False {
          n98 = for {
            N: w230 -> [_]
            tunnel: w228 -> [w250]
            tunnel: w232 -> [w236]
            tunnel: w231 -> [w249]
            tunnel: [w238] -> w227 mode=indexing
            tunnel: w229 -> [w239]
            tunnel: [w234] -> w226 mode=indexing
            tunnel: w225 -> [w233] mode=indexing
            i -> [w248]
            n99 = Quotient & Remainder(x=w248, y=2) -> (x-y*floor(x/y)=w246:i32)  [unwired: 1 out]
            n100 = Not Equal To 0?(x=w246) -> (x != 0?=w241:bool)
            n101 = And(x=w239, y=w241) -> (x .and. y?=w240:bool)
            n102 = Select(t=w236, s=w240, f=sgl 0.0 ("t")) -> (s? t:f=w244:sgl)
            n103 = Add(x=sgl 0.0, y=w244) -> (x+y=w243:sgl)
            n104 = case shown="Default" w249 {
              tunnel: w250 -> [w258 w271]
              tunnel: w236 -> [_ w268]
              tunnel: w249 -> [w257 w265]
              tunnel: w243 -> [_ w263]
              tunnel: [w256 w259] -> w238
              frame 1 {
                n105 = Initialize Array(w258, w257) -> (w256:sgl[])
              }
              frame Default {
                n106 = Divide(x=w271, y=w265) -> (x/y=w269:sgl)
                n107 = expression code="x/2"(w268) -> (w270:sgl)
                n108 = Add(x=w269, y=w270) -> (x+y=w264:sgl)
                n109 = Add(x=w269, y=w268) -> (x+y=w267:sgl)
                n110 = Add(x=w264, y=w263) -> (x+y=w262:sgl)
                n111 = Subtract(x=w264, y=w263) -> (x-y=w260:sgl)
                n112 = expression code="x-2"(w265) -> (w266:u8)
                n113 = for {
                  N: w266 -> [_]
                  tunnel: w267 -> [w272]
                  tunnel: [w272] -> w261 mode=indexing
                }
                n114 = Build Array (concatenate)(w262, w261, w260) -> (w259:sgl[])
              }
            }
            n115 = for {
              tunnel: w238 -> [w255] mode=indexing
              shift-right: [w252] -> _
              shift-left: sgl 0.0 -> [w253]
              tunnel: [w253] -> w235 mode=indexing
              tunnel: w236 -> [w251]
              n116 = Add(x=w255, y=w253) -> (x+y=w254:sgl)
              n117 = Subtract(x=w254, y=w251) -> (x-y=w252:sgl)
            }
            n118 = Add(x=w235, y=w233) -> (x+y=w234:sgl[])
          }
        }
        frame True {
          n119 = for {
            N: w278 -> [_]
            tunnel: w276 -> [w289]
            tunnel: w280 -> [w285]
            tunnel: w279 -> [w287]
            tunnel: [w292] -> w275 mode=indexing
            tunnel: w277 -> [_]
            tunnel: [w282] -> w274 mode=indexing
            tunnel: w273 -> [w281] mode=indexing
            n120 = expression code="x-1"(w287) -> (w284:u8)
            n121 = Multiply(x=w284, y=w285) -> (x*y=w290:sgl)
            n122 = Add(x=w290, y=w289) -> (x+y=w288:sgl)
            n123 = Divide(x=w288, y=w287) -> (x/y=w286:sgl)
            n124 = Initialize Array(w286, w287) -> (w292:sgl[])
            n125 = for {
              tunnel: w292 -> [w297] mode=indexing
              shift-right: [w294] -> _
              shift-left: sgl 0.0 -> [w295]
              tunnel: [w295] -> w283 mode=indexing
              tunnel: w285 -> [w293]
              n126 = Add(x=w297, y=w295) -> (x+y=w296:sgl)
              n127 = Subtract(x=w296, y=w293) -> (x-y=w294:sgl)
            }
            n128 = Add(x=w283, y=w281) -> (x+y=w282:sgl[])
          }
        }
      }
      n129 = case shown="False" w40 {
        tunnel: w115 -> [w141 w177]
        tunnel: w41 -> [w140 w176]
        tunnel: w114 -> [w139 w175]
        tunnel: w113 -> [w138 w174]
        tunnel: w112 -> [w137 w173]
        tunnel: w111 -> [w136 w172]
        tunnel: w110 -> [w135 w171]
        tunnel: [w134 w170] -> w109
        frame True {
          n130 = for {
            N: w140 -> [_]
            tunnel: w136 -> [w145]
            tunnel: w137 -> [w146]
            tunnel: w138 -> [_] mode=indexing
            tunnel: w139 -> [w148]
            tunnel: [w147] -> w134 mode=indexing
            tunnel: w141 -> [_]
            tunnel: w135 -> [w142]
            n131 = expression code="x/2"(w145) -> (w144:sgl)
            n132 = Subtract(x=w142, y=w144) -> (x-y=w143:sgl)
            n133 = case shown="Default" w148 {
              tunnel: w145 -> [_ w159]
              tunnel: w146 -> [_ w160]
              tunnel: w148 -> [w152 w157]
              tunnel: [w151 w154] -> w147
              tunnel: w143 -> [_ w161]
              tunnel: w142 -> [w150 _]
              frame 1 {
                n134 = To Single Precision Float(number=w150) -> (single precision float=w149:sgl)
                n135 = Initialize Array(w149, w152) -> (w151:sgl[])
              }
              frame Default {
                n136 = expression code="x-1"(w157) -> (w166:u8)
                n137 = expression code="x*2"(w157) -> (w163:u8)
                n138 = Multiply(x=w166, y=w160) -> (x*y=w164:sgl)
                n139 = Add(x=w159, y=w164) -> (x+y=w165:sgl)
                n140 = Divide(x=w165, y=w163) -> (x/y=w162:sgl)
                n141 = Subtract(x=w159, y=w160) -> (x-y=w158:sgl)
                n142 = Divide(x=w158, y=w157) -> (x/y=w156:sgl)
                n143 = To Single Precision Float(number=w161) -> (single precision float=w153:sgl)
                n144 = for {
                  N: w157 -> [_]
                  tunnel: w156 -> [w168]
                  tunnel: [w167] -> w155 mode=indexing
                  i -> [w169]
                  n145 = Multiply(x=w168, y=w169) -> (x*y=w167:sgl)
                }
                n146 = Compound Arithmetic op=ADD(w153, w162, w155) -> (w154:sgl[])
              }
            }
          }
        }
        frame False {
          n147 = for {
            N: w176 -> [_]
            tunnel: w172 -> [w185]
            tunnel: w173 -> [w191]
            tunnel: w174 -> [w178] mode=indexing
            tunnel: w175 -> [w196]
            tunnel: [w179] -> w170 mode=indexing
            tunnel: w177 -> [w186]
            tunnel: w171 -> [w182]
            i -> [w195]
            n148 = expression code="x/2"(w185) -> (w184:sgl)
            n149 = Quotient & Remainder(x=w195, y=2) -> (x-y*floor(x/y)=w193:i32)  [unwired: 1 out]
            n150 = Subtract(x=w182, y=w184) -> (x-y=w183:sgl)
            n151 = Not Equal To 0?(x=w193) -> (x != 0?=w188:bool)
            n152 = And(x=w186, y=w188) -> (x .and. y?=w187:bool)
            n153 = Select(t=w191, s=w187, f=sgl 0.0 ("t")) -> (s? t:f=w190:sgl)
            n154 = Add(x=sgl 0.0, y=w190) -> (x+y=w189:sgl)
            n155 = case shown="Default" w196 {
              tunnel: w185 -> [_ w205]
              tunnel: w191 -> [_ w216]
              tunnel: w196 -> [w199 w214]
              tunnel: w189 -> [_ w202]
              tunnel: [w198 w208] -> w180
              tunnel: w183 -> [_ w211]
              tunnel: w182 -> [w197 _]
              frame 1 {
                n156 = Initialize Array(w197, w199) -> (w198:sgl[])
              }
              frame Default {
                n157 = Divide(x=w205, y=w214) -> (x/y=w203:sgl)
                n158 = expression code="x/2"(w216) -> (w217:sgl)
                n159 = Add(x=w203, y=w217) -> (x+y=w213:sgl)
                n160 = To Single Precision Float(number=w211) -> (single precision float=w200:sgl)
                n161 = Add(x=w213, y=w202) -> (x+y=w212:sgl)
                n162 = Subtract(x=w213, y=w202) -> (x-y=w207:sgl)
                n163 = expression code="x-2"(w214) -> (w215:u8)
                n164 = expression code="x/2"(w212) -> (w210:sgl)
                n165 = expression code="x/2"(w207) -> (w204:sgl)
                n166 = for {
                  N: w215 -> [_]
                  tunnel: w203 -> [w224]
                  tunnel: w202 -> [w222]
                  tunnel: [w221] -> w201 mode=indexing
                  i -> [w218]
                  n167 = Add(x=sgl 1.5, y=w218) -> (x+y=w219:sgl)
                  n168 = Multiply(x=w224, y=w219) -> (x*y=w223:sgl)
                  n169 = Add(x=w223, y=w222) -> (x+y=w221:sgl)
                }
                n170 = Subtract(x=w205, y=w204) -> (x-y=w206:sgl)
                n171 = Build Array (concatenate)(w210, w201, w206) -> (w209:sgl[])
                n172 = Add(x=w200, y=w209) -> (x+y=w208:sgl[])
              }
            }
            n173 = Add(x=w180, y=w178) -> (x+y=w179:sgl[])
          }
        }
      }
      "X center (um)" <- w109
      n174 = expression code="x/1000"(w125) -> (w117:sgl)
      n175 = Index Array(array=w98) -> (element #1=w96:bool, element #2=w97:bool)  [unwired: 2 in]
      n176 = Index Array(array=w92) -> (element #1=w94:bool, element #2=w93:bool)  [unwired: 2 in]
      n177 = Index Array(array=w87) -> (element #1=w85:bool, element #2=w86:bool)  [unwired: 2 in]
      n178 = Index Array(array=w82) -> (element #1=w84:bool, element #2=w83:bool)  [unwired: 2 in]
      n179 = Index Array(array=w79) -> (element #1=w77:bool, element #2=w78:bool)  [unwired: 2 in]
      n180 = And(x=w96, y=w97) -> (x .and. y?=w95:bool)
      n181 = And(x=w94, y=w93) -> (x .and. y?=w89:bool)
      n182 = And(x=w85, y=w86) -> (x .and. y?=w69:bool)
      n183 = And(x=w84, y=w83) -> (x .and. y?=w71:bool)
      n184 = And(x=w77, y=w78) -> (x .and. y?=w70:bool)
      n185 = case shown="True" w95 {
        tunnel: w133 -> [w401 w405]
        tunnel: w73 -> [w404 _]
        tunnel: w72 -> [w403 _]
        tunnel: [w402 w405] -> w132
        tunnel: w67 -> [w398 _]
        frame False {
          n186 = Reshape Array(w401, w398) -> (w400:sgl[])
          n187 = call-poly <vilib>:"Mean.vi"("X"=w400) -> ("mean"=w399:dbl)  [unwired: 1 out]
          n188 = Initialize Array(w399, w404, w403) -> (w402:dbl[][])
        }
        frame True {
        }
      }
      n189 = case shown="False" w89 {
        tunnel: w90 -> [w391 w397]
        tunnel: w73 -> [w396 _]
        tunnel: w72 -> [w395 _]
        tunnel: [w394 w397] -> w130
        tunnel: w62 -> [w390 _]
        frame False {
          n190 = Reshape Array(w391, w390) -> (w393:sgl[])
          n191 = call-poly <vilib>:"Mean.vi"("X"=w393) -> ("mean"=w392:dbl)  [unwired: 1 out]
          n192 = Initialize Array(w392, w396, w395) -> (w394:dbl[][])
        }
        frame True {
        }
      }
      n193 = case shown="False" w69 {
        tunnel: w76 -> [w383 w389]
        tunnel: w73 -> [w388 _]
        tunnel: w72 -> [w387 _]
        tunnel: [w386 w389] -> w129
        tunnel: w61 -> [w382 _]
        frame False {
          n194 = Reshape Array(w383, w382) -> (w385:sgl[])
          n195 = call-poly <vilib>:"Mean.vi"("X"=w385) -> ("mean"=w384:dbl)  [unwired: 1 out]
          n196 = Initialize Array(w384, w388, w387) -> (w386:dbl[][])
        }
        frame True {
        }
      }
      n197 = case shown="False" w71 {
        tunnel: w75 -> [w375 w381]
        tunnel: w73 -> [w380 _]
        tunnel: w72 -> [w379 _]
        tunnel: [w378 w381] -> w128
        tunnel: w60 -> [w374 _]
        frame False {
          n198 = Reshape Array(w375, w374) -> (w377:sgl[])
          n199 = call-poly <vilib>:"Mean.vi"("X"=w377) -> ("mean"=w376:dbl)  [unwired: 1 out]
          n200 = Initialize Array(w376, w380, w379) -> (w378:dbl[][])
        }
        frame True {
        }
      }
      n201 = case shown="False" w70 {
        tunnel: w74 -> [w368 w373]
        tunnel: w73 -> [w372 _]
        tunnel: w72 -> [w371 _]
        tunnel: [w370 w373] -> w101
        tunnel: w59 -> [w366 _]
        frame False {
          n202 = Reshape Array(w368, w366) -> (w367:sgl[])
          n203 = call-poly <vilib>:"Mean.vi"("X"=w367) -> ("mean"=w369:dbl)  [unwired: 1 out]
          n204 = Initialize Array(w369, w372, w371) -> (w370:dbl[][])
        }
        frame True {
        }
      }
      n205 = Bundle By Name(cluster=w54, "SEM Scan Parameters.X stig"=w132, "SEM Scan Parameters.Y stig"=w130, "SEM Scan Parameters.X aln"=w129, "SEM Scan Parameters.Y aln"=w128, "SEM Scan Parameters.WD (mm)"=w101) -> (w131:T6)
      n206 = local write "Tiled scan inputs"(w131) -> ()
      n207 = Transpose 2D Array(2D array=w102) -> (transposed array=→"Y center (um)":sgl[][])
      n208 = Transpose 2D Array(2D array=w47) -> (transposed array=w46:sgl[][])
      n209 = Transpose 2D Array(2D array=w119) -> (transposed array=w53:sgl[][])
      n210 = Divide(x=w49, y=w117) -> (x/y=→"X resolution":sgl[][])
      n211 = Multiply(x=w49, y=w56) -> (x*y=→"X size (V)":dbl[][])
      n212 = Divide(x=w53, y=w117) -> (x/y=→"Y resolution":sgl[][])
      n213 = Divide(x=w48, y=w52) -> (x/y=→"Tiled image X index":sgl[][])
      n214 = Divide(x=w46, y=w52) -> (x/y=→"Tiled image Y index":sgl[][])
    }
    frame #2 {
      n215 = local read "Tiled scan inputs"() -> (w407:T6)
      n216 = Unbundle By Name(w407) -> ("SEM Scan Parameters.Frames"=w406:u8)
      n217 = for {
        N: w406 -> [_]
        tunnel: w407 -> [w422]
        i -> [w421]
        stop <- w420 stop-if-true
        # "Frame"
        n218 = Unbundle By Name(w422) -> ("SEM Options"=w451:T7, "HW Config"=w450:T8, "Det Info"=w449:T9, "SEM Scan Parameters"=w464:T10, "Focus Index Options"=w413:T11, "File Information"=w448:T12, "Milling para"=w444:T13)
        n219 = Unbundle By Name(w422) -> ("SEM Options.Detector A"=w432:bool, "SEM Options.Detector B"=w431:bool)
        n220 = Unbundle By Name(w464) -> ("X stig"=w456:sgl[][], "Y stig"=w455:sgl[][], "X aln"=w454:sgl[][], "Y aln"=w453:sgl[][], "Scan rate (Hz)"=w463:u32, "Oversampling"=w462:u32, "Oversampling auto"=w461:bool, "Frame line rampdown ratio"=w460:sgl, "Pixel size (nm)"=w459:sgl, "WD (mm)"=w452:sgl[][])
        n221 = Unbundle By Name(w413) -> ("Keep aspect ratio"=w408:bool, "X Grids"=w412:u8[][], "Y Grids"=w411:u8[][], "Primary X index"=w410:u8[][], "Primary Y index"=w409:u8[][])
        n222 = local read "X resolution"() -> (w458:u32[][])
        n223 = local read "Y resolution"() -> (w457:u32[][])
        n224 = local read "X center (um)"() -> (w447:sgl[][])
        n225 = local read "Y center (um)"() -> (w446:sgl[][])
        n226 = local read "X size (V)"() -> (w445:dbl[][])
        n227 = for {
          tunnel: w463 -> [w509]
          tunnel: w462 -> [w508]
          tunnel: w461 -> [w507]
          tunnel: w460 -> [w506]
          tunnel: w459 -> [w505]
          tunnel: w458 -> [w504] mode=indexing
          tunnel: w457 -> [w503] mode=indexing
          tunnel: w456 -> [w502] mode=indexing
          tunnel: w455 -> [w501] mode=indexing
          tunnel: w454 -> [w500] mode=indexing
          tunnel: w453 -> [w499] mode=indexing
          tunnel: w452 -> [w498] mode=indexing
          tunnel: w451 -> [w497]
          tunnel: w450 -> [w496]
          tunnel: w449 -> [w495]
          tunnel: w448 -> [w494]
          tunnel: w447 -> [w493] mode=indexing
          tunnel: w446 -> [w492] mode=indexing
          tunnel: w445 -> [w491] mode=indexing
          tunnel: w444 -> [w490]
          tunnel: [w488] -> w437 mode=indexing
          tunnel: [w487] -> w436 mode=indexing
          tunnel: [w486] -> w435 mode=indexing
          tunnel: [w485] -> w434 mode=indexing
          tunnel: [w484] -> w440 mode=indexing
          tunnel: [w483] -> w439 mode=indexing
          tunnel: [w482] -> w443 mode=indexing
          tunnel: [w481] -> w442 mode=indexing
          tunnel: [w480] -> w433 mode=indexing
          tunnel: w432 -> [w479]
          tunnel: w431 -> [w478]
          tunnel: [w477] -> w426 mode=concatenating
          tunnel: w421 -> [w476]
          tunnel: [w475] -> w419 mode=indexing
          tunnel: [w474] -> w418 mode=indexing
          tunnel: [w473] -> w414 mode=indexing
          tunnel: [w472] -> w415 mode=indexing
          tunnel: [w471] -> w416 mode=indexing
          tunnel: [w470] -> w417 mode=indexing
          tunnel: w412 -> [w469] mode=indexing
          tunnel: w411 -> [w468] mode=indexing
          tunnel: w410 -> [w467] mode=indexing
          tunnel: w409 -> [w466] mode=indexing
          tunnel: w408 -> [w465]
          i -> [w489]
          # "Y"
          n228 = for {
            tunnel: w509 -> [w572]
            tunnel: w508 -> [w571]
            tunnel: w507 -> [w570]
            tunnel: w506 -> [w569]
            tunnel: w505 -> [w535]
            tunnel: w504 -> [w529] mode=indexing
            tunnel: w503 -> [w528] mode=indexing
            tunnel: w502 -> [w568] mode=indexing
            tunnel: w501 -> [w567] mode=indexing
            tunnel: w500 -> [w566] mode=indexing
            tunnel: w499 -> [w565] mode=indexing
            tunnel: w498 -> [w538] mode=indexing
            tunnel: w497 -> [w553]
            tunnel: w496 -> [w559]
            tunnel: w495 -> [w558]
            tunnel: w494 -> [w556]
            tunnel: w493 -> [w564] mode=indexing
            tunnel: w492 -> [w563] mode=indexing
            tunnel: w491 -> [w539] mode=indexing
            tunnel: w490 -> [w555]
            tunnel: w489 -> [w534]
            tunnel: [w550] -> w488 mode=indexing
            tunnel: [w549] -> w487 mode=indexing
            tunnel: [w548] -> w486 mode=indexing
            tunnel: [w547] -> w485 mode=indexing
            tunnel: [w545] -> w484 mode=indexing
            tunnel: [w544] -> w483 mode=indexing
            tunnel: [w543] -> w482 mode=indexing
            tunnel: [w542] -> w481 mode=indexing
            tunnel: [w532] -> w480 mode=indexing
            tunnel: w479 -> [w531]
            tunnel: w478 -> [w530]
            tunnel: [w527] -> w477 mode=indexing
            tunnel: w476 -> [w526]
            tunnel: [w524] -> w475 mode=indexing
            tunnel: [w521] -> w474 mode=indexing
            tunnel: [w520] -> w473 mode=indexing
            tunnel: [w519] -> w472 mode=indexing
            tunnel: [w518] -> w471 mode=indexing
            tunnel: [w517] -> w470 mode=indexing
            tunnel: w469 -> [w514] mode=indexing
            tunnel: w468 -> [w513] mode=indexing
            tunnel: w467 -> [w512] mode=indexing
            tunnel: w466 -> [w511] mode=indexing
            tunnel: w465 -> [w510]
            i -> [w533]
            # "X"
            n229 = shared-variable ".\\Zeiss Library.lvlib\\X resolution"(w529) -> ()  [unwired: 1 in, 1 out]
            n230 = Build Array(w534, w533) -> (w552:i32[])
            n231 = Bundle By Name(cluster="SEM Scan Parameters", "X resolution"=w529, "Y resolution"=w528, "X center (um)"=w564, "Y center (um)"=w563, "X size (V)"=w539, "X size auto"=FALSE, "X stig"=w568, "Y stig"=w567, "X aln"=w566, "Y aln"=w565, "Scan rate (Hz)"=w572, "Oversampling"=w571, "Oversampling auto"=w570, "Frame line rampdown ratio"=w569, "Pixel size (nm)"=w535, "WD (mm)"=w538) -> (w557:T5)
            n232 = Bundle By Name(cluster="Focus Index Options", "Keep aspect ratio"=w510, "X Grids"=w514, "Y Grids"=w513, "Primary X index"=w512, "Primary Y index"=w511) -> (w515:T1)
            n233 = flat-sequence {
              tunnel: w534 -> [w581]
              tunnel: w533 -> [w580]
              tunnel: w532 -> [w586]
              tunnel: w531 -> [w574]
              tunnel: w530 -> [w573]
              frame #0 {
                n234 = local read "Det A Img Tiled"() -> (w591:i16[][])
                n235 = shared-variable ".\\Zeiss Library.lvlib\\Det A Img"() -> (w588:i16[][])  [unwired: 1 in, 1 out]
                n236 = shared-variable ".\\Zeiss Library.lvlib\\Det B Img"() -> (w585:i16[][])  [unwired: 1 in, 1 out]
                n237 = local read "Tiled image scale (um/pix)"() -> (w587:sgl)
                n238 = local read "Tiled image Y index"() -> (w593:u16[][])
                n239 = local read "Tiled image X index"() -> (w592:u16[][])
                n240 = local read "Det B Img Tiled"() -> (w582:i16[][])
                n241 = Index Array(array=w593, index (row)=w581, index (col)=w580) -> (element=w578:u16)
                n242 = Index Array(array=w592, index (row)=w581, index (col)=w580) -> (element=w577:u16)
                n243 = Divide(x=w586, y=w587) -> (x/y=w579:dbl)
                n244 = call "2D Array Zoom.vi"("y zoom factor"=w579, "x zoom factor"=w579, "Input 2D Array"=w588) -> ("output array"=w590:dbl[][])  [unwired: 6 in, 2 out]
                n245 = call "2D Array Zoom.vi"("y zoom factor"=w579, "x zoom factor"=w579, "Input 2D Array"=w585) -> ("output array"=w583:dbl[][])  [unwired: 6 in, 2 out]
                n246 = To Word Integer(number=w590) -> (16bit integer=w589:i16[][])
                n247 = To Word Integer(number=w583) -> (16bit integer=w584:i16[][])
                n248 = Replace Array Subset(array=w591, new element=w589, index (row)=w578, index (col)=w577) -> (w575:i16[][])
                n249 = Replace Array Subset(array=w582, new element=w584, index (row)=w578, index (col)=w577) -> (w576:i16[][])
                n250 = case shown="True" w574 {
                  tunnel: w575 -> [_ w595]
                  frame False {
                  }
                  frame True {
                    n251 = local write "Det A Img Tiled"(w595) -> ()
                    n252 = shared-variable ".\\Zeiss Library.lvlib\\Det A Img Tiled"(w595) -> ()  [unwired: 1 in, 1 out]
                  }
                }
                n253 = case shown="True" w573 {
                  tunnel: w576 -> [_ w594]
                  frame False {
                  }
                  frame True {
                    n254 = shared-variable ".\\Zeiss Library.lvlib\\Det B Img Tiled"(w594) -> ()  [unwired: 1 in, 1 out]
                    n255 = local write "Det B Img Tiled"(w594) -> ()
                  }
                }
              }
            }
            n256 = shared-variable ".\\Zeiss Library.lvlib\\Y resolution"(w528) -> ()  [unwired: 1 in, 1 out]
            n257 = call "2D scan Tclk.vi"("HW Config"=w559, "Options"=w553, "Frame"=w526, "Det Info"=w558, "Scan Para"=w557, "Focus Index Options"=w515, "File Info"=w556, "Tile index"=w552, "Milling para"=w555) -> ("Image Focus Index Array"=w546:T14, "Info & Status"=w523:T15, "SEM parameters"=w522:T16, "8-bit over scale"=w527:bool[], "FIB parameters"=w554:T17, "Image Focus Index"=w551:T18)  [unwired: 1 in]
            n258 = Unbundle By Name(w546) -> ("A Img Focus Index array"=w545:sgl[][], "B Img Focus Index array"=w544:sgl[][], "C Img Focus Index array"=w543:sgl[][], "D Img Focus Index array"=w542:sgl[][])
            n259 = Unbundle By Name(w522) -> ("Working distance"=w521:sgl, "Stig X"=w520:sgl, "Stig Y"=w519:sgl, "Alignment X"=w518:sgl, "Alignment Y"=w517:sgl)
            n260 = Unbundle By Name(w551) -> ("A Img Focus Index"=w550:sgl, "B Img Focus Index"=w549:sgl, "C Img Focus Index"=w548:sgl, "D Img Focus Index"=w547:sgl)
            n261 = Unbundle By Name(w523) -> ("Decimating factor"=w540:u16)
            n262 = local read "Single scan outputs"() -> (w561:T4)
            n263 = Bundle By Name(cluster=w561, "Image Focus Index Array"=w546, "SEM Status"=w523, "SEM Parameters"=w522, "FIB parameters"=w554, "Image Focus Index"=w551) -> (w525:T4)
            "Single scan outputs" <- w525
            n264 = expression code="x/1000"(w535) -> (w537:sgl)
            n265 = Quotient & Remainder(x=w529, y=w540) -> (floor(x/y)=w541:u32)  [unwired: 1 out]
            n266 = Divide(x=w529, y=w541) -> (x/y=w536:dbl)
            n267 = Unbundle By Name(w525) -> ("SEM Status.SEM Spec. I (nA)"=w524:sgl)
            n268 = Multiply(x=w537, y=w536) -> (x*y=w532:dbl)
          }
        }
        "Low res scale Tiled (um/pix)" <- w433
        "SEM Spec. I Tiled (nA)" <- w419
        "WD Tiled" <- w418
        "Stig X Tiled" <- w414
        "Stig Y Tiled" <- w415
        "Aln X Tiled" <- w416
        "Aln Y Tiled" <- w417
        n269 = Bundle("A Img Focus Index array"=w440, "B Img Focus Index array"=w439, "C Img Focus Index array"=w443, "D Img Focus Index array"=w442) -> (→"Image Focus Index Array Tiled":T2)  [unwired: 1 in]
        n270 = Bundle(w437, w436, w435, w434) -> (→"Image Focus Index Tiled":cluster{sgl[][], sgl[][], sgl[][], sgl[][]})  [unwired: 1 in]
        n271 = Index Array(array=w426, index (col) #1=0 ("index (row)"), index (col) #2=1 ("index (row)")) -> (element #1=w427:bool[], element #2=w428:bool[])  [unwired: 2 in]
        n272 = And Array Elements(Boolean array=w427) -> (logical AND=w425:bool)
        n273 = And Array Elements(Boolean array=w428) -> (logical AND=w423:bool)
        n274 = Build Array(w425, w423) -> (→"8-bit over scale":bool[])
        n275 = shared-variable "My Computer\\Zeiss Library.lvlib\\Stop"() -> (w420:bool)  [unwired: 1 in, 1 out]
      }
    }
    frame #3 {
      n276 = shared-variable "My Computer\\Zeiss Library.lvlib\\Machine Type"() -> (w596:u8)  [unwired: 1 in, 1 out]
      n277 = case shown="2" w596 {
        frame 0, Default {
          n278 = local read "Tiled scan inputs"() -> (w598:T6)
          n279 = Unbundle By Name(w598) -> ("HW Config.Eanable COM"=w597:bool)
          n280 = case shown="True" w597 {
            tunnel: w598 -> [_ w614]
            frame False {
            }
            frame True {
              n281 = Unbundle By Name(w614) -> ("HW Config.COM port"=w613:refnum<visa-resource-name>, "SEM Scan Parameters.Y tiles"=w612:u8, "SEM Scan Parameters.X tiles"=w611:u8)  [unwired: 5 out]
              n282 = local read "Stig X Tiled"() -> (w603:sgl[][])
              n283 = local read "Stig Y Tiled"() -> (w602:sgl[][])
              n284 = expression code="(x-1)/2"(w612) -> (w606:u8)
              n285 = expression code="(x-1)/2"(w611) -> (w605:u8)
              n286 = Index Array(array=w603, index (row)=w606, index (col)=w605) -> (element=w610:sgl)
              n287 = Index Array(array=w602, index (row)=w606, index (col)=w605) -> (element=w609:sgl)
              n288 = Format Into String(format string="stim %g %g", w610, w609) -> (resulting string=w626:string)  [unwired: 2 in, 1 out]
              n289 = local read "Aln X Tiled"() -> (w601:sgl[][])
              n290 = local read "Aln Y Tiled"() -> (w600:sgl[][])
              n291 = call "Remcon32 command.vi"("Initialization"=TRUE, "SEM command"=w626, "COM port in"=w613) -> ("error out"=w617:errorcluster, "COM port out"=w618:refnum<visa-resource-name>)  [unwired: 2 in, 5 out]
              n292 = Index Array(array=w601, index (row)=w606, index (col)=w605) -> (element=w608:sgl)
              n293 = Index Array(array=w600, index (row)=w606, index (col)=w605) -> (element=w607:sgl)
              n294 = Format Into String(format string="aaln %g %g", w608, w607) -> (resulting string=w624:string)  [unwired: 2 in, 1 out]
              n295 = local read "WD Tiled"() -> (w599:sgl[][])
              n296 = call "Remcon32 command.vi"("error in"=w617, "SEM command"=w624, "COM port in"=w618) -> ("error out"=w615:errorcluster, "COM port out"=w616:refnum<visa-resource-name>)  [unwired: 2 in, 5 out]
              n297 = Index Array(array=w599, index (row)=w606, index (col)=w605) -> (element=w604:sgl)
              n298 = Format Into String(format string="focs %g", w604) -> (resulting string=w622:string)  [unwired: 2 in, 1 out]
              n299 = call "Remcon32 command.vi"("Close session"=TRUE, "error in"=w615, "SEM command"=w622, "COM port in"=w616) -> ()  [unwired: 1 in, 7 out]
            }
          }
        }
        frame 2 {
          n300 = local read "Tiled scan inputs"() -> (w655:T6)
          n301 = invoke class="_EMApi" method="InitialiseRemoting"(reference="Api") -> (reference out=w634:refnum<k7>)  [unwired: 2 in, 2 out]
          n302 = Unbundle By Name(w655) -> ("SEM Scan Parameters.Y tiles"=w654:u8, "SEM Scan Parameters.X tiles"=w653:u8)  [unwired: 5 out]
          n303 = local read "Stig X Tiled"() -> (w650:sgl[][])
          n304 = local read "Stig Y Tiled"() -> (w649:sgl[][])
          n305 = expression code="(x-1)/2"(w654) -> (w652:u8)
          n306 = expression code="(x-1)/2"(w653) -> (w651:u8)
          n307 = Index Array(array=w650, index (row)=w652, index (col)=w651) -> (element=w633:sgl)
          n308 = Index Array(array=w649, index (row)=w652, index (col)=w651) -> (element=w627:sgl)
          n309 = local read "Aln X Tiled"() -> (w648:sgl[][])
          n310 = local read "Aln Y Tiled"() -> (w647:sgl[][])
          n311 = call "SmartSEM Remote API set float.vi"("vValue"=w633, "lpszParam"="AP_STIG_X" ("lpszCommand"), "Api"=w634) -> ("error out"=w641:errorcluster, "Api out"=w642:refnum<k7>)  [unwired: 7 in]
          n312 = call "SmartSEM Remote API set float.vi"("vValue"=w627, "lpszParam"="AP_STIG_Y" ("lpszCommand"), "Api"=w634) -> ("error out"=w630:errorcluster, "Api out"=w631:refnum<k7>)  [unwired: 7 in]
          n313 = Index Array(array=w648, index (row)=w652, index (col)=w651) -> (element=w639:sgl)
          n314 = Index Array(array=w647, index (row)=w652, index (col)=w651) -> (element=w628:sgl)
          n315 = local read "WD Tiled"() -> (w646:sgl[][])
          n316 = call "SmartSEM Remote API set float.vi"("error in"=w641, "vValue"=w639, "lpszParam"="AP_APERTURE_ALIGN_X" ("lpszCommand"), "Api"=w642) -> ("error out"=w637:errorcluster, "Api out"=w638:refnum<k7>)  [unwired: 6 in]
          n317 = call "SmartSEM Remote API set float.vi"("error in"=w630, "vValue"=w628, "lpszParam"="AP_APERTURE_ALIGN_Y" ("lpszCommand"), "Api"=w631) -> ()  [unwired: 6 in, 2 out]
          n318 = Index Array(array=w646, index (row)=w652, index (col)=w651) -> (element=w645:sgl)
          n319 = expression code="x/1000"(w645) -> (w635:sgl)
          n320 = call "SmartSEM Remote API set float.vi"("error in"=w637, "vValue"=w635, "lpszParam"="AP_WD" ("lpszCommand"), "Api"=w638) -> ()  [unwired: 6 in, 2 out]
        }
      }
    }
  }
